vi "STC_main_raw_dev_MQTTT_RT_raw.vi"() -> ()   [LabVIEW 2017]
uses:
  controls/FPGA State.ctl
  mqtt Folder/src/class/mqtt/mqttTypedef/mqttConnectionStatus.ctl
  mqtt Folder/src/class/mqtt/mqttTypedef/mqttConnectionMeta.ctl
  mqtt Folder/src/class/mqtt/mqttTypedef/mqttQOSlevel.ctl
  controls/UI Data2.ctl
  mqtt Folder/src/class/mqtt/mqttTXqueue/mqttTXdataQueueFunction.ctl
  mqtt Folder/src/class/mqtt/mqttConfigFunction.ctl
  mqtt Folder/src/class/mqtt/mqttTypedef/mqttConnectionFlags.ctl
  mqtt Folder/src/class/mqtt/mqttTypedef/mqttWillInformation.ctl
  mqtt Folder/src/class/mqtt/mqttTypedef/mqttBroker.ctl
  controls/Chatter data.ctl
  Globals/Global - All UI Loop Stop.vi
  Globals/Global - UI Stream and Variable Connections.vi
  Globals/Global - Configuration Options.vi
  UI Error Handlers/support/User Event - Stop/User Event - Stop.lvlib
  UI Error Handlers/support/Message Queue/Message Queue.lvlib
  mqtt Folder/src/class/mqtt/mqtt.lvclass
panel:
  out "publishSuccess":bool=TRUE
  out "publishMessageID":u16 format="%02x"
  in  "connMeta":T1
  in  "topic":string="a/b"
  out "connStatus 2":T3
  out "success":bool
  out "sessionPresent 2":bool
  in  "error in (no error)":errorcluster
  out "tag acc":string
  out "tag spike":string
  out "string":string
  out "x .or. y?":bool
  out "resulting string":string
  out "Raw Waveform":waveform(dbl)[](graph)
  in  "Settings Tab":T4(tab)=enum."Data Monitoring"
  in  "Database_machine":string="Raw.Starrag_STC_1250_V1"
  in  "OK Button":bool
  in  "Tool Data File":path=path "K:/Core Research/Project Folders/AI Projects/AI3190 Digital Shop Floor Rollout/5 Software Files/Catapult/tool_path.txt"
  in  "Run Control":bool
  in  "Stop Control":bool
  in  "Max Acceleration Threshold (g)":sgl=0.03
  in  "In-cut Power Threshold":dbl=1.0
  in  "Controller Address":string="143.167.158.195"
  in  "Connect to Controller":bool
  out "Connected?":bool
  out "System Status":string
  in  "Save?":bool
  in  "Switch to Safe State":bool
  out "Current FPGA State":T5
  out "Tool Data":string="\n"
  in  "ODBC data source name":string="amrc_monitoring"
  in  "MT Connect Agent":string="http://amrcmtconnect.shef.ac.uk:5000/"
  in  "milliseconds to wait":u32=100
  in  "Machine":string="STC1250"
  out "Loop execution":u32
  out "output cluster":cluster{"G1 ":bool}
  out "Chatter?":bool
  out "Feed":dbl
  out "ACC  (grms)":T6(graph)
  out "Block of code being executed":string
  out "Program Name":string
  out "RPM":dbl
  out "STC Starrag":bool
  out "Force (grms)":T7(graph)
  out "Tool id":string
  out "Spindle Load":dbl[](graph)
  out "CPU Usage (%)":dbl[][](graph)
  out "Free Physical Memory or Largest Contiguous Memory (bytes)":dbl(graph)
  out "DMA FIFO Overflow?":bool
  in  "Exit":bool
  # "Acceleration Waveform for 0.5s"
  # "Connection Settings"
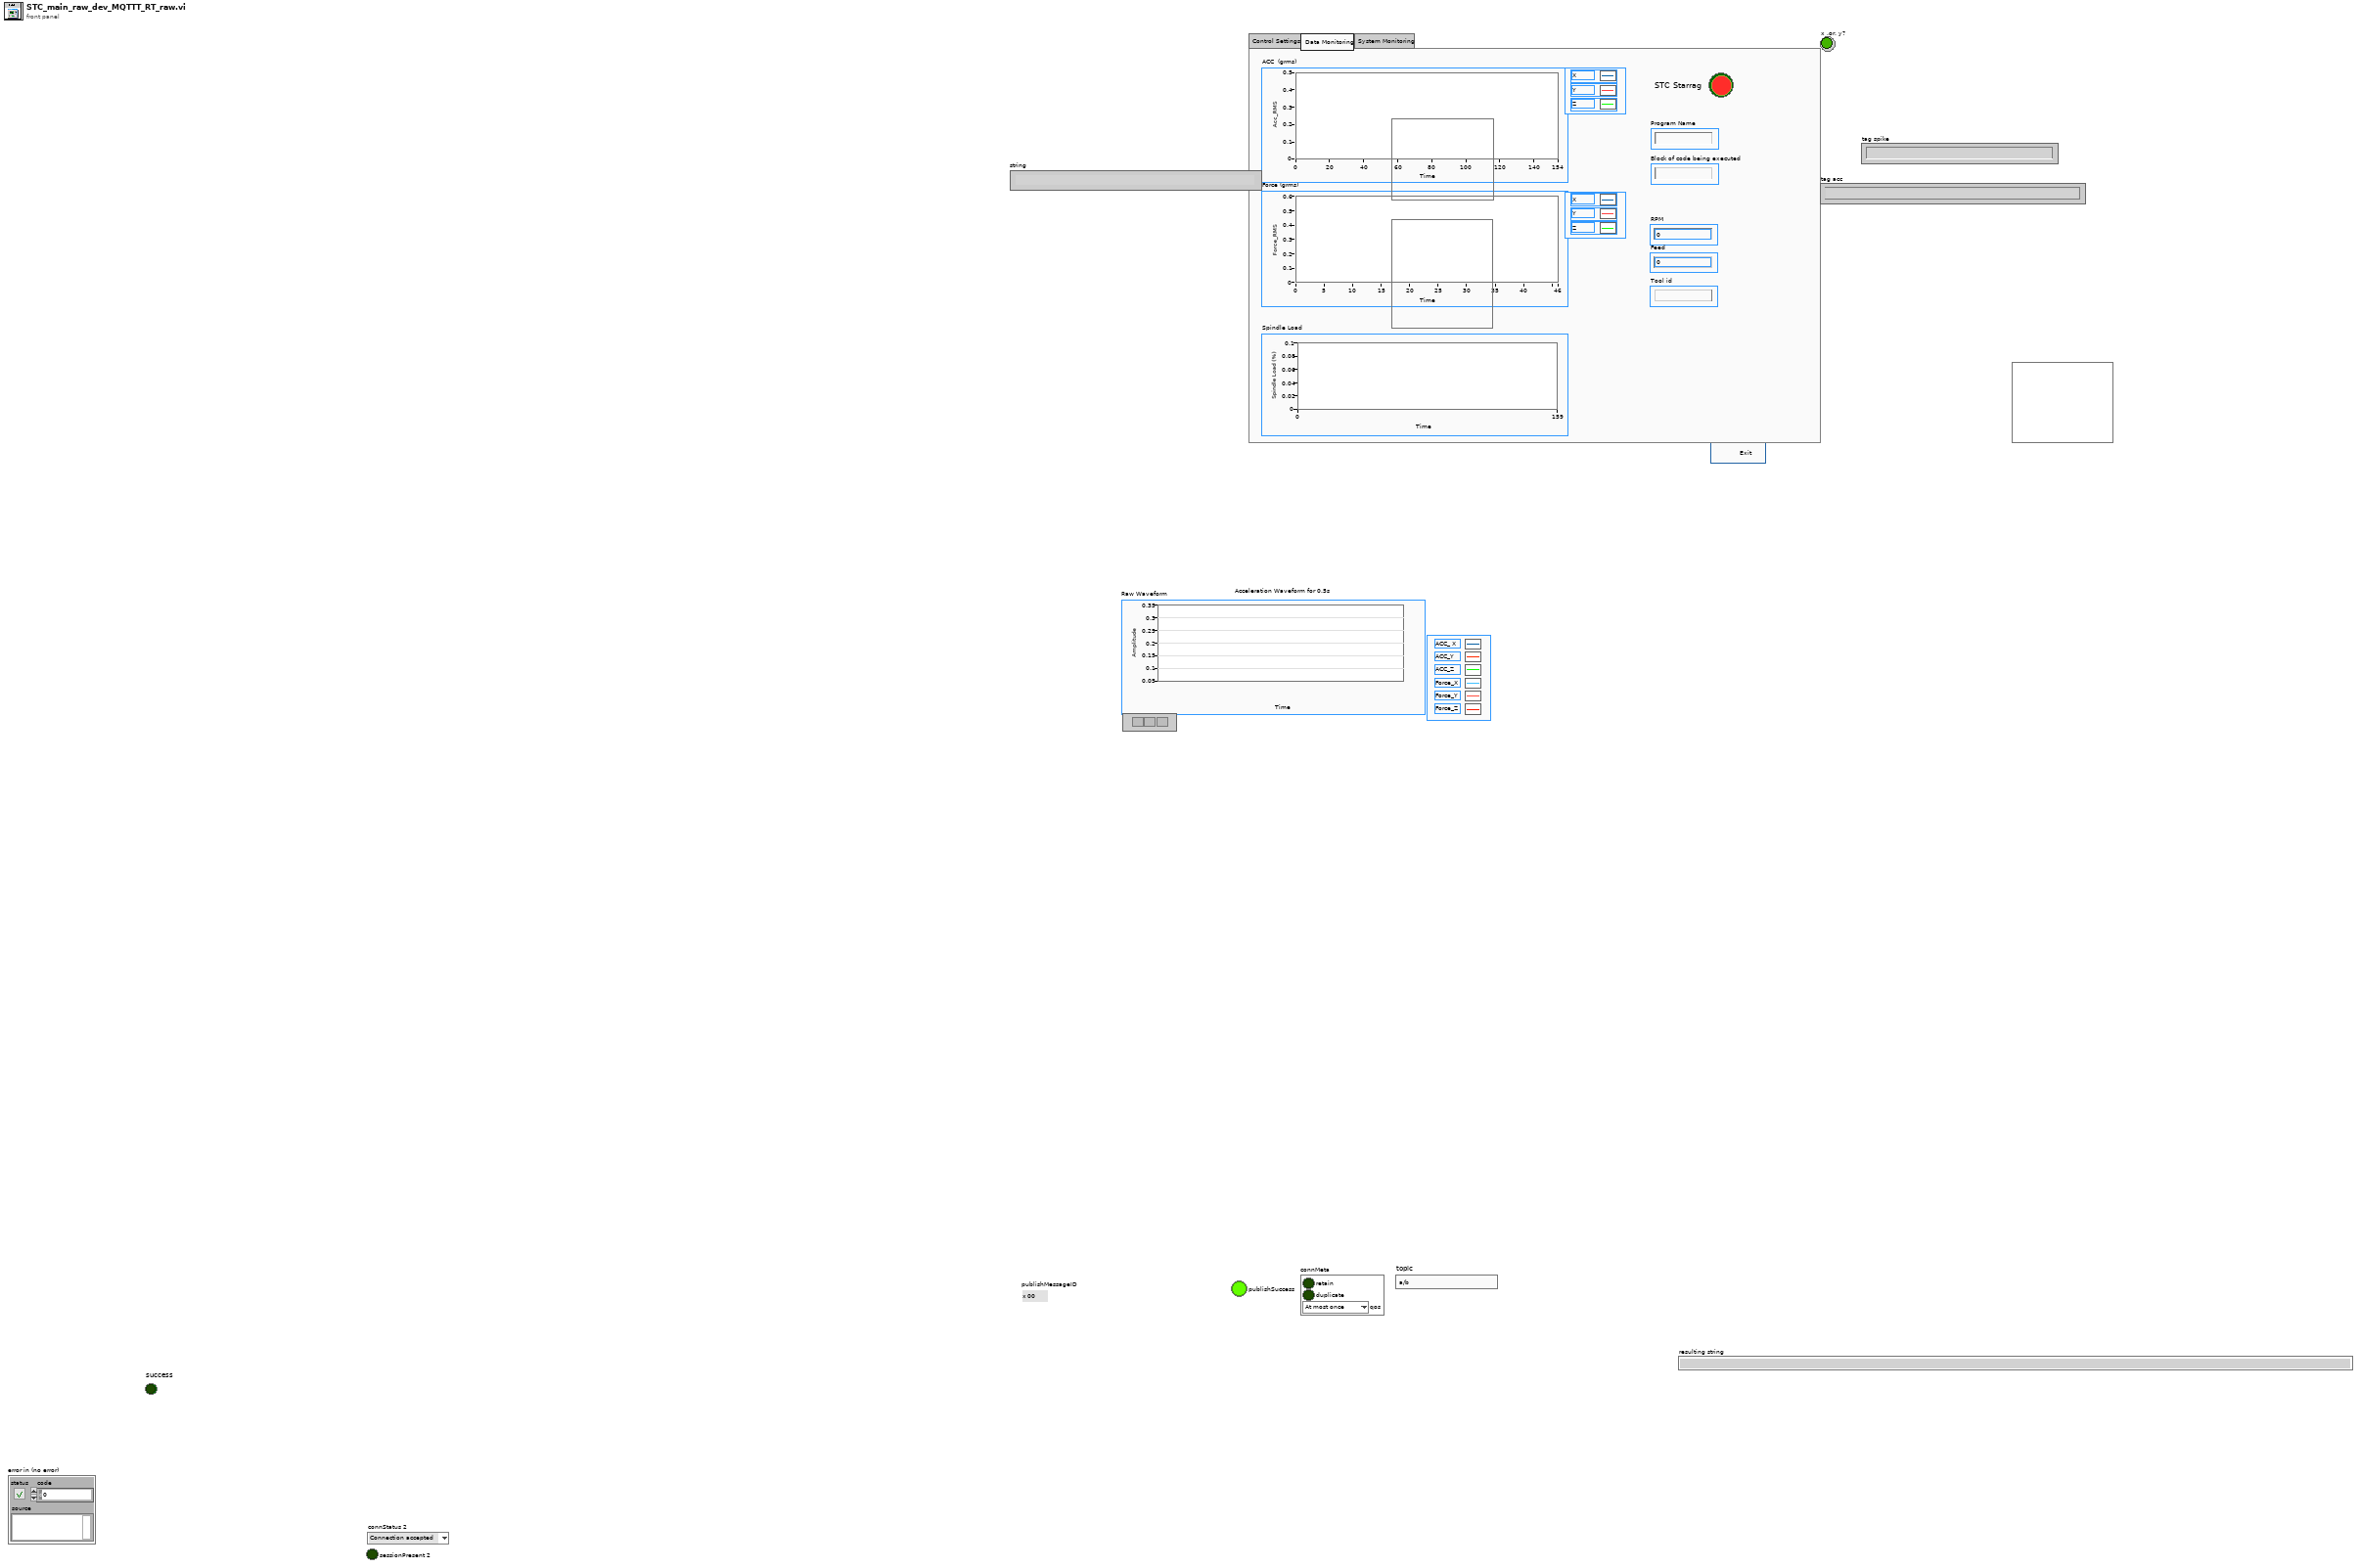
[diagram p1: front panel]
types:
  T1 = typedef "mqttConnectionMeta.ctl" = cluster{"retain":bool, "duplicate":bool, "qos":T2}
  T2 = typedef "mqttQOSlevel.ctl" = enum8{"At most once", "At least once", "Exactly once", "Reserved"}
  T3 = typedef "mqttConnectionStatus.ctl" = enum16{"Connection accepted", "Connection refused: unacceptable protocol version", "Connection refused: identifier rejected", "Connection refused: Server unavailable", "Connection refused: bad user name or password", "Connection refused: not authorized"}
  T4 = enum32{"Control Settings", "Data Monitoring", "System Monitoring"}
  T5 = typedef "FPGA State.ctl" = enum16{"Safe State", "Control (PID)"}
  T6 = cluster{"Array of Double[0]":dbl, "Array of Double[1]":dbl, "Array of Double[2]":dbl}
  T7 = cluster{"[0]":dbl, "[1]":dbl, "[2]":dbl, "[3]":dbl, "[4]":dbl, "[5]":dbl, "[6]":dbl, "[7]":dbl}
  T8 = typedef "mqttBroker.ctl" = cluster{"address":string, "port":u16, "connTimeout":i32, "writeTimeout":i32, "readTimeout":i32, "subTimeout":i32}
  T9 = typedef "mqttWillInformation.ctl" = cluster{"User Name":string, "Password":string}
  T10 = typedef "mqttConnectionFlags.ctl" = cluster{"reserved":bool, "clean session":bool, "will flag":bool, "willQOS":enum8{"At most once", "At least once", "Exactly once", "Reserved"}, "will retain":bool, "password":bool, "user name":bool}
  T11 = typedef "mqtt.lvclass/mqttConfigFunction.ctl" = enum16{"init", "deinit", "set", "get"}
  T12 = enum8{"Enabled", "Disabled", "Disabled and Grayed Out"}
  T13 = typedef "mqttTXdataQueueFunction.ctl" = enum16{"init", "deinit", "getQueue", "enqueue"}
  T14 = typedef "UI Data2.ctl" = cluster{"Switch to Safe State Ref":refnum<vi>, "Run Control Ref":refnum<vi>, "Stop Control Ref":refnum<vi>, "Update Control Configurations Ref":refnum<vi>, "Chatter Data Ref":refnum<vi>, "Max Acceleration Threshold Ref":refnum<vi>}
  T15 = typedef "Message Queue.lvlib/All Message Queues.ctl" = cluster{"UI":refnum<queue>}
  T16 = cluster{"Message":string, "Message Data":variant}
  T17 = typedef "Chatter data.ctl" = cluster{"Tool data":cluster{"Number of teeth":sgl}, "Cutting data":cluster{"rpm":sgl}, "Limits":cluster{"Magnitude threshold":sgl, "Tolerance":sgl}, "G1 status":cluster{"G1 ":bool}}
  T18 = cluster{"FPGA State":T5, "Max Acceleration Threshold":sgl, "Chatter Data":T17}
  T19 = cluster{"seconds since 1Jan1904":timestamp, "number":dbl[][], "Machine Data":cluster{"Zload":string, "Yload":string, "Xload":string, "path_position":string, "Fovr":string, "SspeedOvr":string, "Program Name":string, "Program status":string, "Block of code being executed":string, "Line of code":string, "Machine availability":string, "Emergency status":string, "Controller mode":string, "Tool_id":string}}
  T20 = cluster{"seconds since 1Jan1904":timestamp, "number":dbl[][], "Machine Data":cluster{"Zload":string, "Yload":string, "Xload":string, "path_position":string, "Fovr":string, "SspeedOvr":string, "Program Name":string, "Program status":string, "Block of code being executed":string, "Line of code":string, "Machine availability":string, "Emergency status":string, "Controller mode":string, "Tool id":string}}
  T21 = cluster{"Actual PID Loop Period":refnum<k21>, "DMA FIFO Overflow?":refnum<k21>, "CPU Usage":refnum<k21>, "Free or Contiguous Memory":refnum<k21>, "Current FPGA State":refnum<k21>, "Acceleration (grms)":refnum<k21>, "Acceleration Waveform":refnum<k21>, "Chatter":refnum<k21>, "tag acc":refnum<k21>, "tag video":refnum<k21>, "Image Waveform":refnum<k21>}
  T22 = cluster{"Zload":string, "Yload":string, "Xload":string, "path_position":string, "Fovr":string, "SspeedOvr":string, "Program Name":string, "Program status":string, "Block of code being executed":string, "Line of code":string, "Machine availability":string, "Emergency status":string, "Controller mode":string, "Tool_id":string}
  T23 = cluster{"Zload":string, "Yload":string, "Xload":string, "path_position":string, "Fovr":string, "SspeedOvr":string, "Program Name":string, "Program status":string, "Block of code being executed":string, "Line of code":string, "Machine availability":string, "Emergency status":string, "Controller mode":string, "Tool id":string}
  T24 = cluster{"Magnitude threshold":sgl, "Tolerance":sgl}
  T25 = typedef "FPGA state.ctl" = enum16{"Safe State", "Control (PID)"}
  T26 = typedef "IMAQ Image.ctl" = refnum<image>
  T27 = typedef "CPU Loads.ctl" = cluster{"Total (%)":dbl, "Time Critical (%)":dbl, "Timed Structures (%)":dbl, "High (%)":dbl, "Above Normal (%)":dbl, "Normal (%)":dbl, "Background (%)":dbl, "Idle (%)":dbl, "ISR (%)":dbl}[]
  T28 = cluster{"seconds since 1Jan1904":timestamp, "appended array":dbl[][], "Machine Data":cluster{"Zload":string, "Yload":string, "Xload":string, "path_position":string, "Fovr":string, "SspeedOvr":string, "Program Name":string, "Program status":string, "Block of code being executed":string, "Line of code":string, "Machine availability":string, "Emergency status":string, "Controller mode":string, "Tool_id":string}}
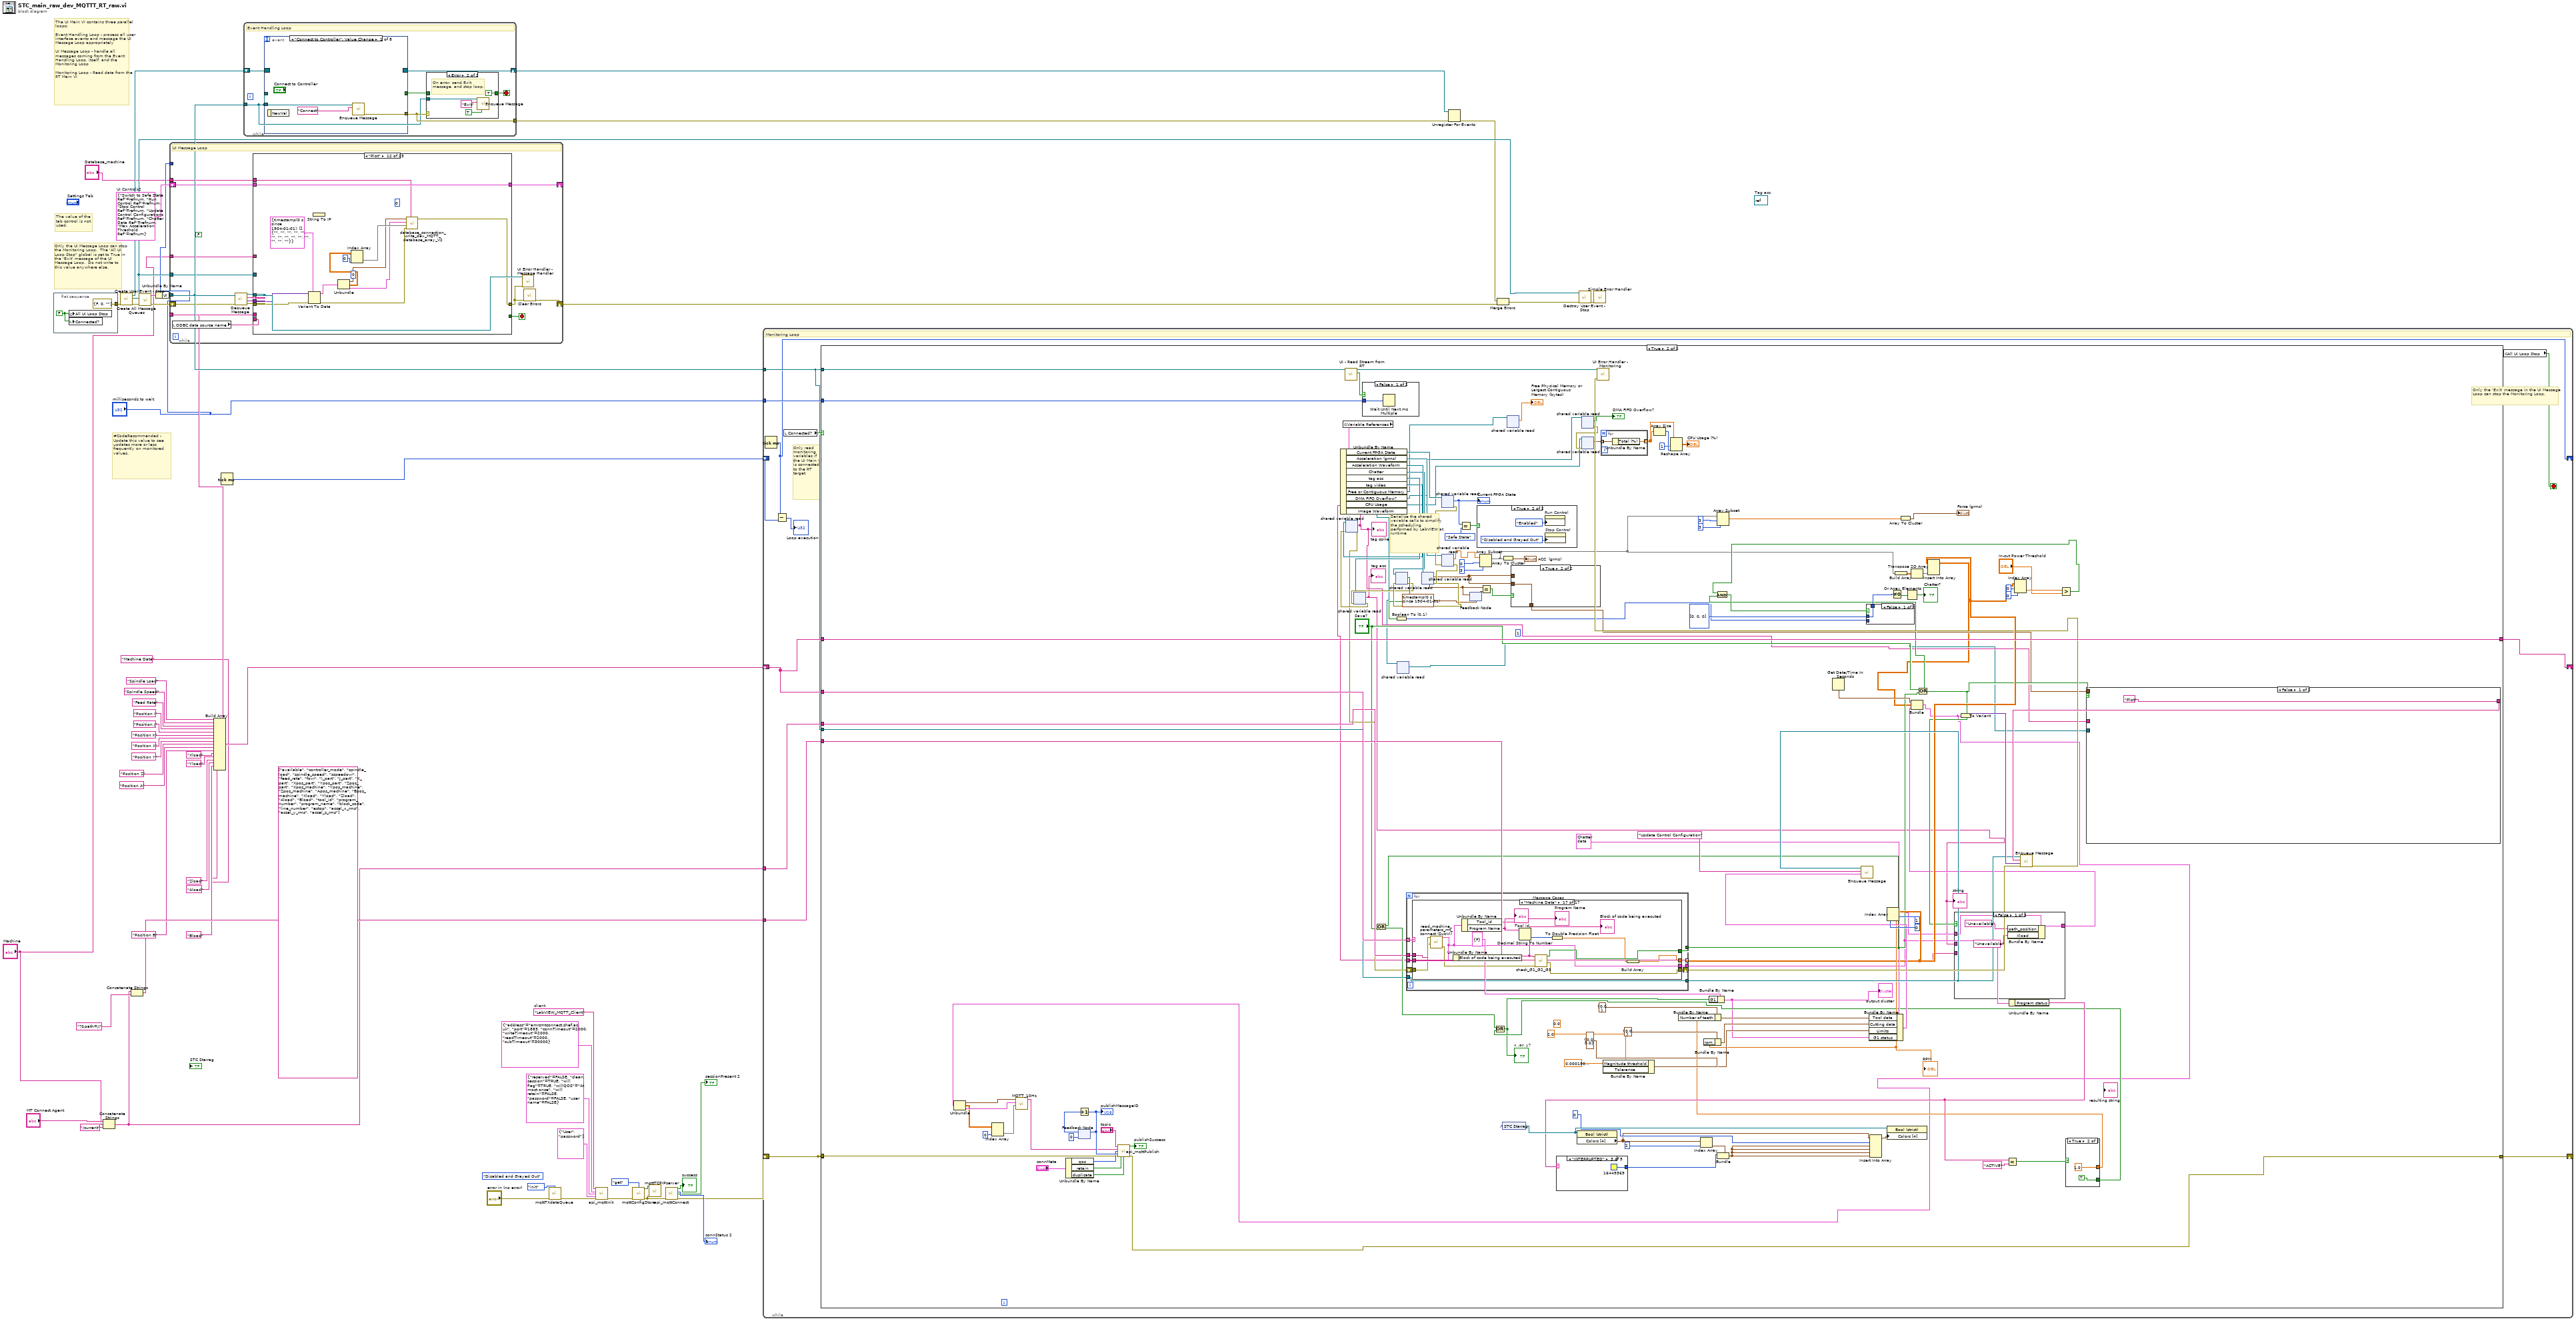
[diagram p0: block diagram]
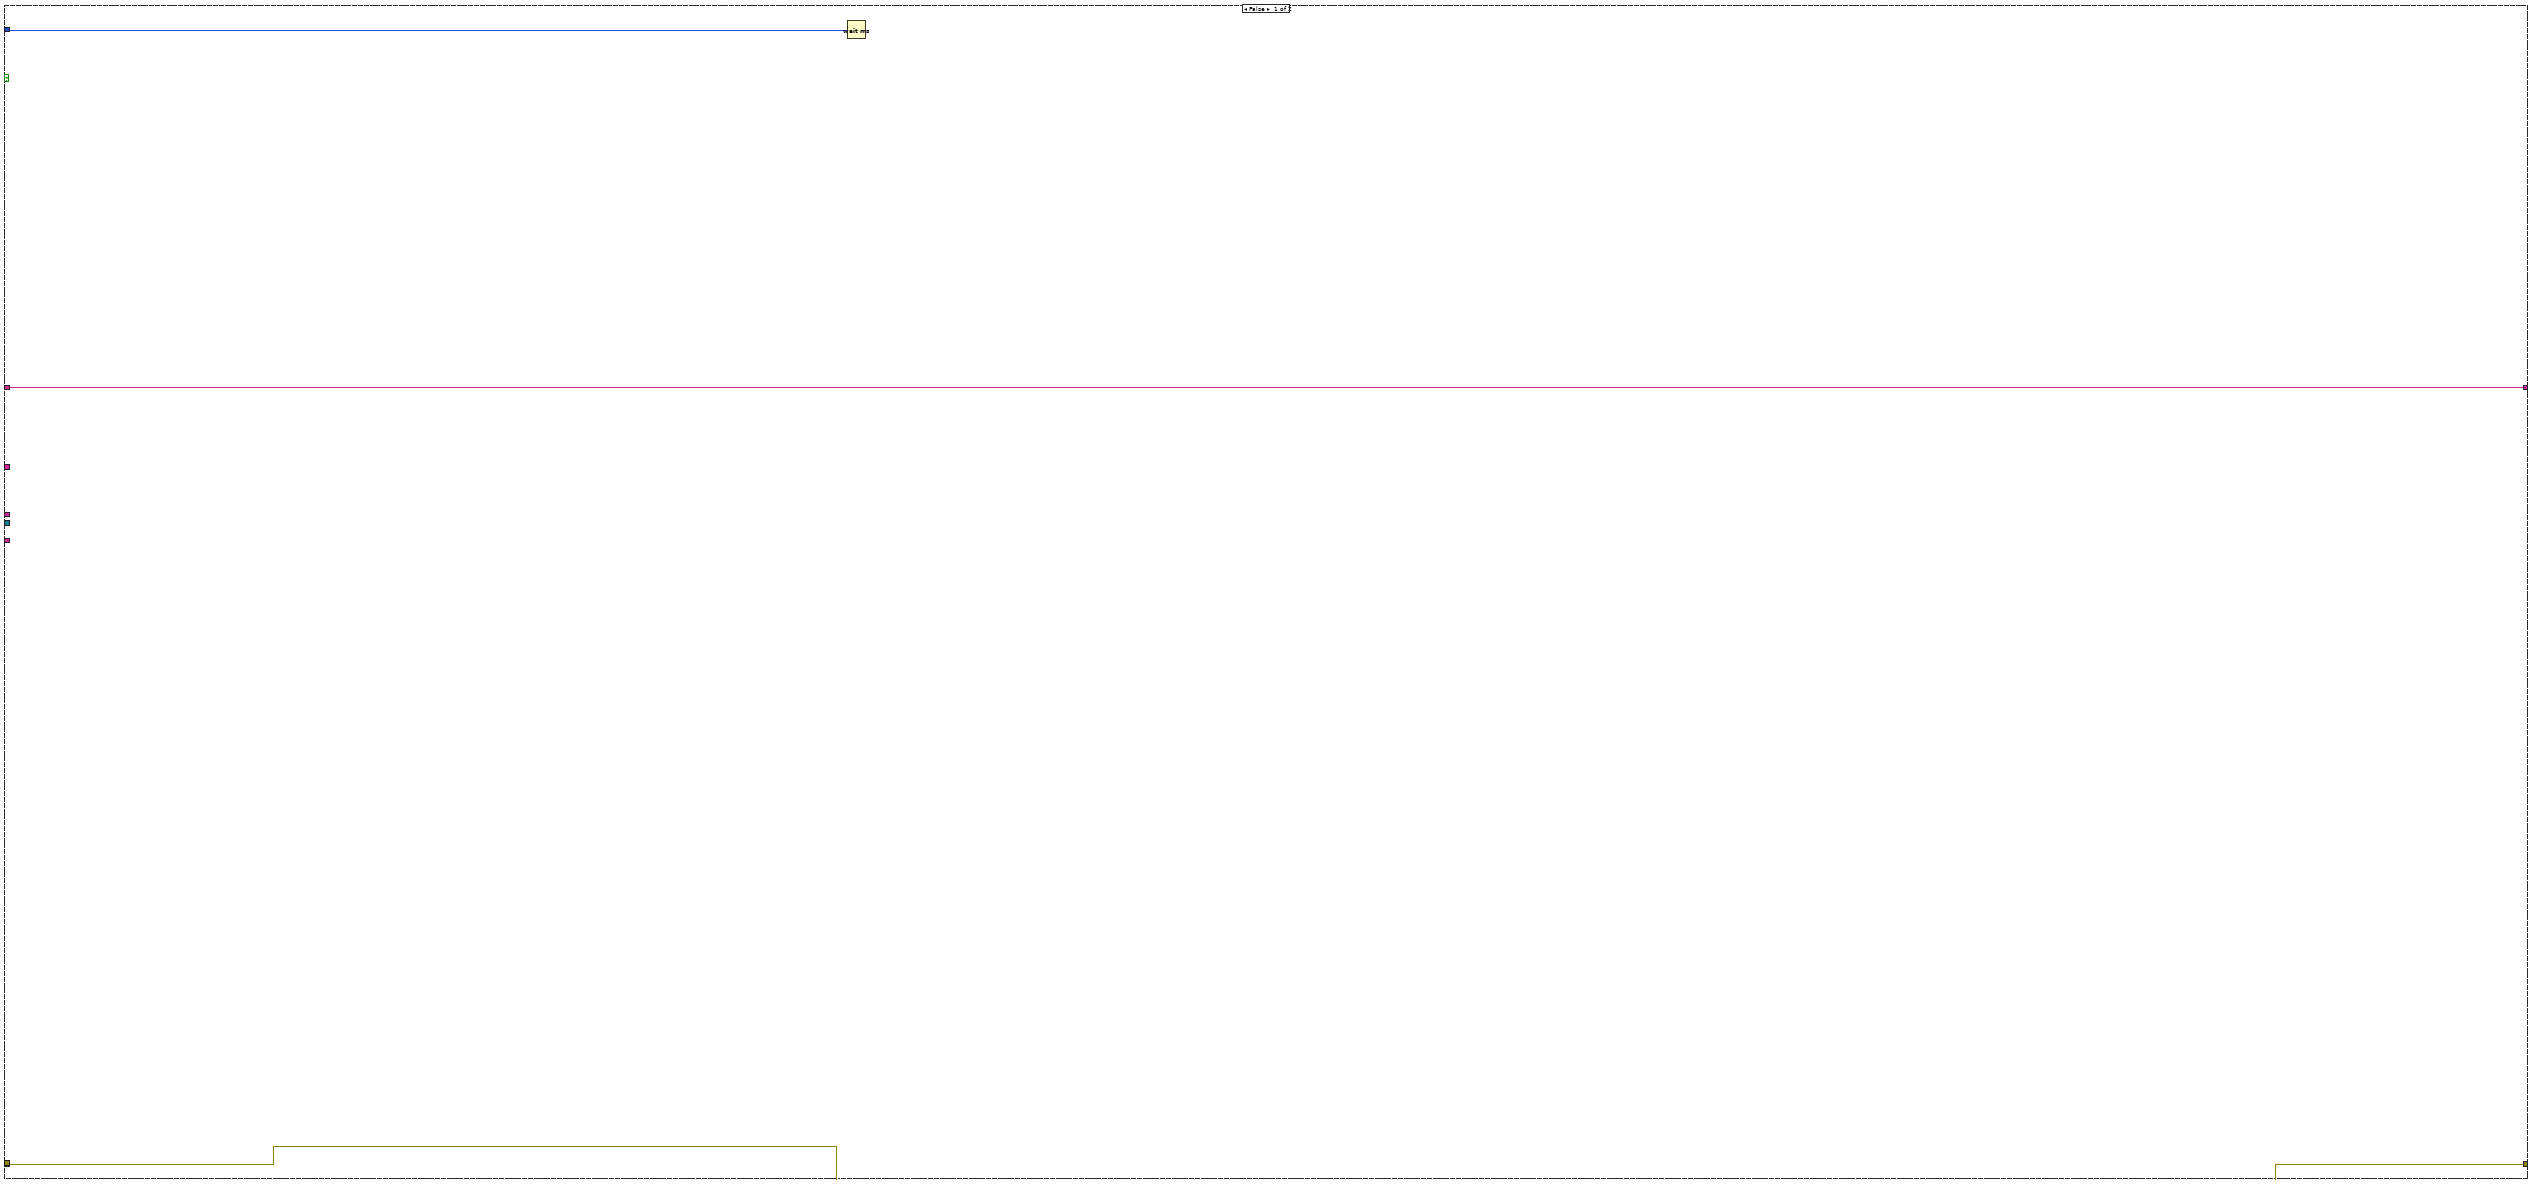
[diagram p2: hidden frame]
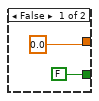
[diagram p3: hidden frame]
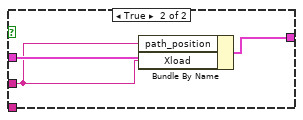
[diagram p4: hidden frame]
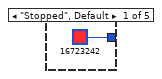
[diagram p5: hidden frame]
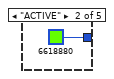
[diagram p6: hidden frame]
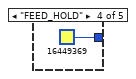
[diagram p7: hidden frame]
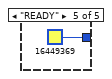
[diagram p8: hidden frame]
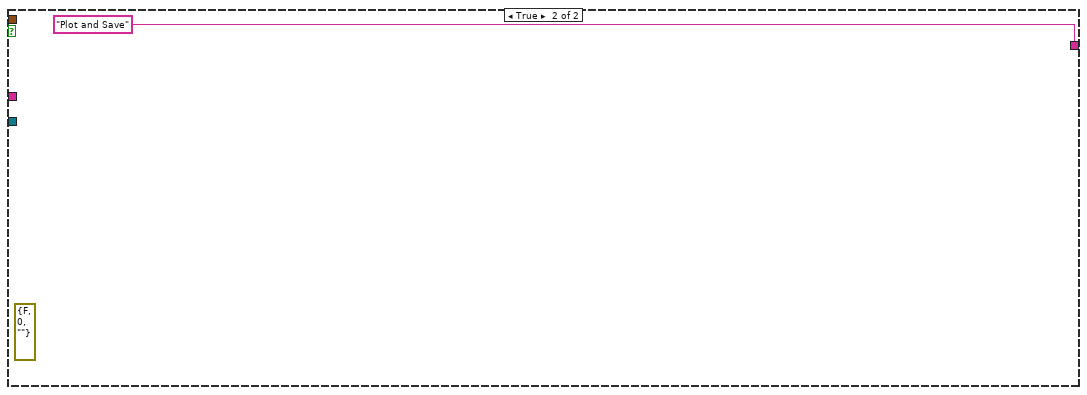
[diagram p10: hidden frame]
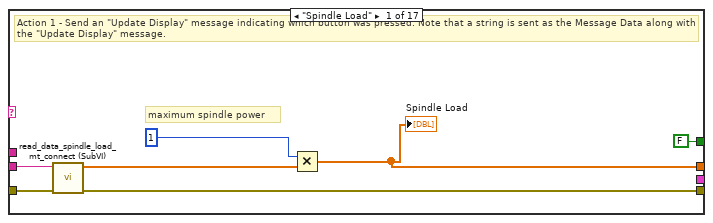
[diagram p11: hidden frame]
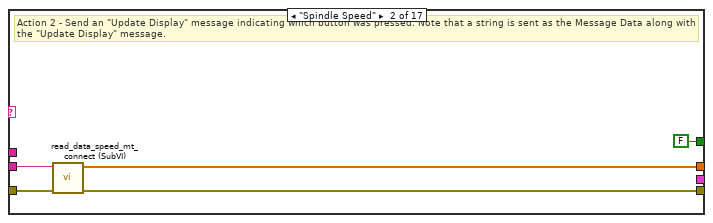
[diagram p12: hidden frame]
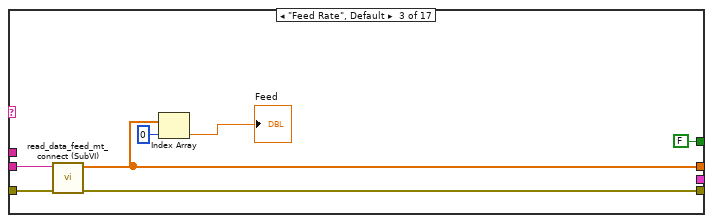
[diagram p13: hidden frame]
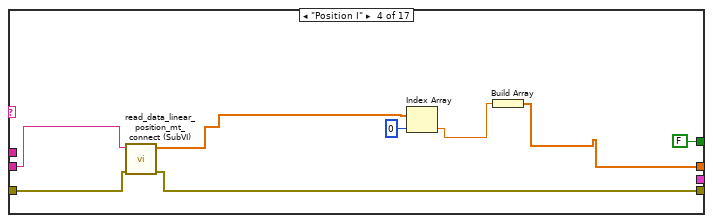
[diagram p14: hidden frame]
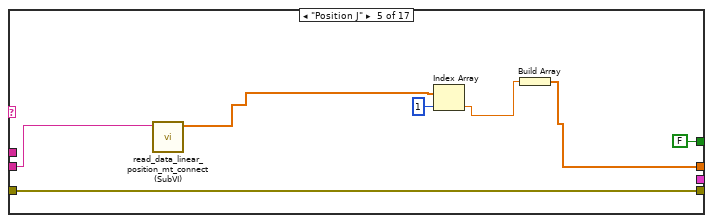
[diagram p15: hidden frame]
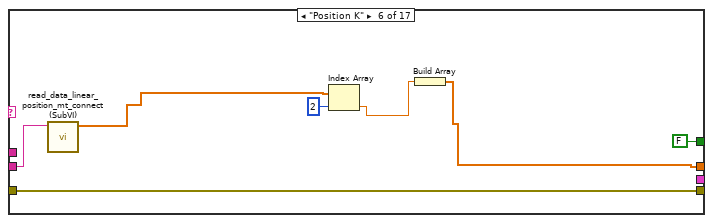
[diagram p16: hidden frame]
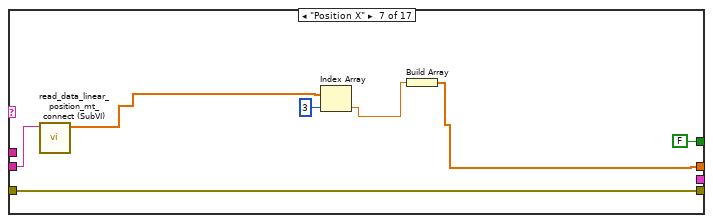
[diagram p17: hidden frame]
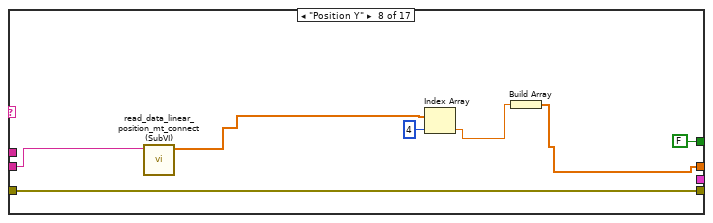
[diagram p18: hidden frame]
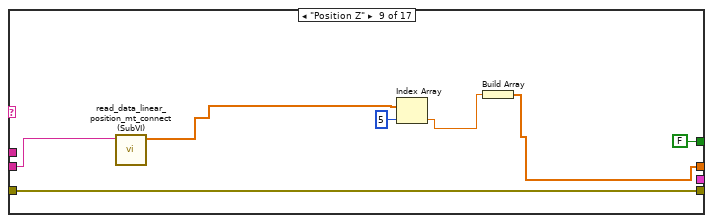
[diagram p19: hidden frame]
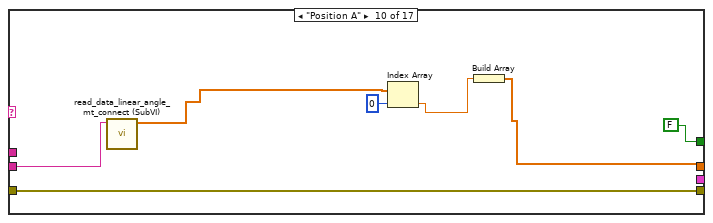
[diagram p20: hidden frame]
diagram:
  w6 = "LabVIEW_MQTT_Client"  # client
  (unwired) T12."Disabled and Grayed Out" ("Disabled")
  (unwired) string[] ["available", "controller_mode", "spindle_load", "spindle_speed", "sspeedovr", "feed_rate", "fovr", "I_part", "J_part", "K_part", "Xpos_part", "Ypos_part", "Zpos_part", "Xpos_machine", "Ypos_machine", "Zpos_machine", "Apos_machine", "Bpos_machine", "Xload", "Yload", "Zload", "Aload", "Bload", "tool_id", "program_number", "program_name", "block_code", "line_number", "estop", "accel_x_rms", "accel_y_rms", "accel_z_rms"]
  (unwired) refnum<k21> refnum  # Tag acc
  (unwired) FALSE ("Record  SS 661")
  w43 = T14 {"Switch to Safe State Ref"=refnum, "Run Control Ref"=refnum, "Stop Control Ref"=refnum, "Update Control Configurations Ref"=refnum, "Chatter Data Ref"=refnum, "Max Acceleration Threshold Ref"=refnum}  # UI Controls2
  # "#CodeRecommended - Update this value to see updates more or less frequently on monitored values."
  # "The UI Main VI contains three parallel loops:\n\nEvent Handling Loop - process all user interface events and message the UI Message Loop appropriately\n\nUI Message Loop - handle all messages coming from the Event Handling Loop, itself, and the Monitoring Loop\n\nMonitoring Loop - Read data from the RT Main VI"
  # "The value of the tab control is not used."
  # "Only the UI Message Loop can stop the Monitoring Loop.  The 'All UI Loop Stop\" global is set to True in the 'Exit' message of the UI Message Loop.  Do not write to this value anywhere else."
  n1 = flat-sequence {
    tunnel: [errorcluster {"status"=FALSE, "code"=0, "source"=""} ("error in (no error)")] -> w44
    frame #0 {
      w57 = FALSE
      n2 = global write "Global - All UI Loop Stop.vi" "All UI Loop Stop"(w57) -> ()
      n3 = local write "Connected?"(w57) -> ()
    }
  }
  n4 = Concatenate Strings("MT Connect Agent", "Machine", "/current" ("string")) -> (w34:string)
  n5 = call "Create User Event - Stop.vi"("error in (no error)"=w44) -> ("error out"=w51:errorcluster, "User Event - Stop"=w52:refnum<user-event>, "Stop Event Registration Refnum"=w53:refnum<event-registration>)  [unwired: 8 in]
  n6 = Concatenate Strings(w34, "?&path=//" ("string")) -> (w38:string)
  n7 = call "Create All Message Queues.vi"("error in (no error)"=w51) -> ("error out"=w49:errorcluster, "Message Queues out"=w50:T15)  [unwired: 9 in]
  n8 = Unbundle By Name(w50) -> ("UI"=w45:refnum<queue>)
  n9 = Build Array("Spindle Load" ("Message"), "Spindle Speed" ("Message"), "Feed Rate" ("element"), "Position I" ("element"), "Position J" ("element"), "Position K" ("element"), "Position X" ("element"), "Position Y" ("element"), "Position Z" ("element"), "Position A" ("element"), "Position B" ("element"), "Xload" ("element"), "Yload" ("element"), "Zload" ("element"), "Aload" ("element"), "Bload" ("element"), "Machine Data" ("element")) -> (w37:string[])
  n10 = while {
    tunnel: w45 -> [w68]
    tunnel: w52 -> [w73]
    shift-right: [w63] -> w56
    shift-left: w49 -> [w72]
    shift-right: [w66] -> _
    shift-left: w43 -> [w67]
    tunnel: w37 -> [w62]
    tunnel: "Machine" -> [w61]
    tunnel: "milliseconds to wait" -> [_]
    tunnel: "Database_machine" -> [w59]
    stop <- w74 stop-if-true
    # "UI Message Loop"
    n11 = local read "ODBC data source name"() -> (w60:string)
    n12 = call "Dequeue Message.vi"("error in (no error)"=w72, "Message Queue"=w68) -> ("error out"=w71:errorcluster, "Message Data"=w69:variant, "Message"=w70:string, "dup Message Queue"=w65:refnum<queue>)  [unwired: 6 in]
    n13 = case "Message Cases" shown="\"Plot\"" w70 {
      selector: w70 -> [_ _ _ _ _ _ _ _ _ _ _ _ w205 _ w239 _ w274 _ _ _ _ _ w373]
      tunnel: w65 -> [w76 w82 _ _ w115 _ w133 w141 _ w166 _ _ w206 _ _ _ w278 _ w321 _ _ w347 _]
      tunnel: w71 -> [w78 w89 w102 w108 w120 w131 w135 w139 w155 w175 w189 w202 w208 w226 w240 w258 w288 w309 w326 w331 w343 w348 _]
      tunnel: [w77 w83 w102 w108 w114 w131 w134 w144 w154 w168 w182 w194 w207 w228 w241 w257 w289 w307 w327 w330 w342 w351 w371] -> w64
      tunnel: [_ _ _ _ _ _ _ _ _ _ _ _ _ _ _ _ _ _ TRUE _ _ _ _] -> w74
      tunnel: w69 -> [_ _ _ _ _ _ _ _ _ w173 w188 w201 _ w225 w238 w256 w286 w306 _ _ w340 _ _]
      tunnel: w73 -> [_ _ _ _ _ _ _ _ _ _ _ _ _ _ _ _ _ _ w325 _ _ _ _]
      tunnel: w67 -> [w79 w88 w101 w110 w119 w130 w137 w145 w156 w171 w190 w203 w209 w229 w242 w255 w290 w308 w323 w329 w341 w350 w369]
      tunnel: [w79 w87 w101 w110 w119 w130 w137 w145 w156 w171 w190 w203 w209 w229 w242 w255 w290 w308 w323 w329 w341 w350 w369] -> w66
      tunnel: w62 -> [_ _ _ _ _ _ _ _ _ _ _ _ _ _ _ _ _ _ _ _ _ _ _]
      tunnel: w60 -> [_ _ _ _ _ _ _ _ _ _ _ _ _ _ _ _ _ _ _ _ _ _ _]
      tunnel: w61 -> [_ _ _ _ _ _ _ _ _ _ _ _ _ _ _ _ _ _ _ _ _ _ _]
      tunnel: w59 -> [_ _ _ _ _ _ _ _ _ _ w178 w191 _ _ _ _ _ _ _ _ _ _ _]
      frame "Initialize" {
        # "Initialize - Send 'Initialize UI Refs' message to get the UI references bundled and initialized appropriately."
        n14 = call "Enqueue Message.vi"("error in (no error)"=w78, "Message"="Initialize UI Refs", "Message Queue"=w76) -> ("error out"=w77:errorcluster)  [unwired: 7 in, 1 out]
      }
      frame "Initialize UI Refs" {
        # "Send a message to disable them all, since there is no connection at the start."
        # "Initialize UI Refs - Bundle up a cluster of references of all UI elements that are programmatically manipulated."
        n15 = control-ref of="Max Acceleration Threshold (g)"() -> (w80:refnum<vi>)
        n16 = control-ref of="Switch to Safe State"() -> (w86:refnum<vi>)
        n17 = control-ref of="Run Control"() -> (w85:refnum<vi>)
        n18 = control-ref of="Stop Control"() -> (w84:refnum<vi>)
        n19 = call "Enqueue Message.vi"("error in (no error)"=w89, "Message"="Disable Controls", "Message Queue"=w82) -> ("error out"=w83:errorcluster)  [unwired: 7 in, 1 out]
        n20 = Bundle By Name(cluster=w88, "Switch to Safe State Ref"=w86, "Run Control Ref"=w85, "Stop Control Ref"=w84, "Max Acceleration Threshold Ref"=w80) -> (w87:T14)
      }
      frame "Disable Controls" {
        w92 = 0
        # "With the control options disabled, the only thing the user can do is Connect. Make sure the IP address string and connect button are enabled."
        # "Disable All Controls - Set all controls in the UI Refs cluster to \"Disabled and Grayed Out\"."
        n21 = Unbundle(w101) -> ("Switch to Safe State Ref"=w100:refnum<vi>, "Run Control Ref"=w99:refnum<vi>, "Stop Control Ref"=w98:refnum<vi>, "Update Control Configurations Ref"=w97:refnum<vi>, "Chatter Data Ref"=w96:refnum<vi>, "Max Acceleration Threshold Ref"=w95:refnum<vi>)
        n22 = Build Array(w100, w99, w98, w97, w96, w95) -> (w94:refnum<vi>[])
        n23 = property on="ODBC data source name" class="Str"("DisabledEnum"=T12."Enabled" ("Disabled")) -> ()  [unwired: 2 in, 2 out]
        n24 = property on="In-cut Power Threshold" class="DigNum (strict)"("DisabledEnum"=T12."Disabled and Grayed Out" ("Disabled")) -> ()  [unwired: 2 in, 2 out]
        n25 = call "Set Enable State on Multiple Controls.vi"("Enable?"=FALSE, "Controls"=w94) -> ()  [unwired: 10 in]
        n26 = property on="Controller Address" class="Str"("DisabledEnum"=w92) -> ()  [unwired: 2 in, 2 out]
        n27 = property on="Connect to Controller" class="Bool"("DisabledEnum"=w92) -> ()  [unwired: 2 in, 2 out]
      }
      frame "Enable Configuration Controls" {
        w111 = 2
        # "Once connected, the user shouldn't be able to change the connection settings unless he gets disconnected."
        # "Enable Configuration Controls - After successful connection, ensure appropriate controls are enabled."
        n28 = Unbundle By Name(w110) -> ("Update Control Configurations Ref"=w109:refnum<vi>, "Max Acceleration Threshold Ref"=w107:refnum<vi>, "Chatter Data Ref"=w106:refnum<vi>, "Switch to Safe State Ref"=w105:refnum<vi>)
        n29 = property on="In-cut Power Threshold" class="DigNum (strict)"("DisabledEnum"=T12."Enabled" ("Disabled")) -> ()  [unwired: 2 in, 2 out]
        n30 = property on="ODBC data source name" class="Str"("DisabledEnum"=T12."Disabled and Grayed Out" ("Disabled")) -> ()  [unwired: 2 in, 2 out]
        n31 = Build Array(w109, w107, w106, w105) -> (w113:refnum<vi>[])
        n32 = call "Set Enable State on Multiple Controls.vi"("Enable?"=TRUE, "Controls"=w113) -> ()  [unwired: 10 in]
        n33 = property on="Controller Address" class="Str"("DisabledEnum"=w111) -> ()  [unwired: 2 in, 2 out]
        n34 = property on="Connect to Controller" class="Bool"("DisabledEnum"=w111) -> ()  [unwired: 2 in, 2 out]
      }
      frame "Connect" {
        # "Connect - Attempt to connect to both streams, and the variables, on the RT target."
        n35 = call "UI - Initiate Connection.vi"("error in (no error)"=w120, "Controller Address"="Controller Address", "Message Queue"=w115) -> ("error out"=w117:errorcluster, "Connected?"=w116:bool)  [unwired: 7 in]
        "Connected?" <- w116
        n36 = case shown="True" w116 {
          tunnel: w117 -> [w121 w125]
          tunnel: w115 -> [_ w124]
          tunnel: [w121 w123] -> w114
          frame False {
          }
          frame True {
            n37 = call "Enqueue Message.vi"("error in (no error)"=w125, "Message"="Enable Configuration Controls", "Message Queue"=w124) -> ("error out"=w123:errorcluster)  [unwired: 7 in, 1 out]
          }
        }
      }
      frame "Close Connections" {
        # "Close Connections - Close the connections shared with the Monitoring Loop."
        n38 = global read "Global - UI Stream and Variable Connections.vi" "UI Command Stream"() -> (w129:refnum<k21>)
        n39 = global read "Global - UI Stream and Variable Connections.vi" "RT Message Stream"() -> (w128:refnum<k21>)
        n40 = global read "Global - UI Stream and Variable Connections.vi" "Variable References"() -> (w126:T21)
        n41 = local write "Connected?"(FALSE ("Connected?")) -> ()
        n42 = Destroy Stream Endpoint(11:w129) -> ()  [unwired: 1 in, 1 out]
        n43 = Destroy Stream Endpoint(11:w128) -> ()  [unwired: 1 in, 1 out]
        n44 = call "Close Variable Connections.vi"("Variable References 2"=w126) -> ()  [unwired: 11 in]
      }
      frame "Disconnect UI" {
        # "Disable Controls"
        # "Disconnect UI - Something has gone wrong with the connection. Reinitialize the UI to its disconnected state."
        n45 = local write "Connected?"(FALSE ("Connected?")) -> ()
        n46 = call "Enqueue Message.vi"("error in (no error)"=w135, "Message"="Reconnect", "Message Queue"=w133) -> ("error out"=w134:errorcluster)  [unwired: 7 in, 1 out]
      }
      frame "Reconnect" {
        # "Disconnect UI - Something has gone wrong with the connection. Reinitialize the UI to its disconnected state."
        n47 = Flush Queue(queue=w141, error in (no error)=w139) -> (queue out=w140:refnum<queue>, error out=w138:errorcluster)  [unwired: 1 out]
        n48 = flat-sequence {
          tunnel: w140 -> [w147]
          tunnel: w138 -> [w148]
          tunnel: [w148] -> w143
          tunnel: [w147] -> w142
          tunnel: w143 -> [w151]
          tunnel: w142 -> [w149]
          tunnel: [w150] -> w144
          frame #0 {
            n49 = Wait Until Next ms Multiple(millisecond multiple=u32 10000) -> ()  [unwired: 1 out]
          }
          frame #1 {
            n50 = call "Enqueue Message.vi"("error in (no error)"=w151, "Message"="Connect", "Message Queue"=w149) -> ("error out"=w150:errorcluster)  [unwired: 7 in, 1 out]
          }
        }
      }
      frame "Get Settings from FPGA" {
        # "Get Settings from FPGA - Send a command to the RT to retrieve all current FPGA Main VI parameter values and send them back to the UI."
        n51 = local read "Connected?"() -> (w153:bool)
        n52 = case shown="True" w153 {
          tunnel: w155 -> [w157 w161]
          tunnel: [w157 w160] -> w154
          frame False {
            # "Don't bother trying to send a message to the RT system if UI Main VI isn't even connected"
          }
          frame True {
            n53 = global read "Global - UI Stream and Variable Connections.vi" "UI Command Stream"() -> (w158:refnum<k21>)
            n54 = shared-variable-write(w158, w161, T16 {"Message"="Send FPGA Configuration to UI", "Message Data"=variant} ("data in")) -> (w160:errorcluster)  [unwired: 1 in, 2 out]
          }
        }
      }
      frame "Initial UI Values" {
        # "Set values of all manual and setpoint controls via reference."
        # "Initial UI Values - These are the current values of the FPGA Main VI's R/W controls. They are used to initialize the panel of UI Main VI upon successful connection to the RT target."
        n55 = Variant To Data(error in=w175, type=T18 {"FPGA State"=enum."Safe State", "Max Acceleration Threshold"=0.0, "Chatter Data"={"Tool data"={"Number of teeth"=2.0}, "Cutting data"={"rpm"=9898.0}, "Limits"={"Magnitude threshold"=0.0, "Tolerance"=1.0}, "G1 status"={"G1 "=FALSE}}}, Variant=w173) -> (data=w172:T18, error out=w174:errorcluster)
        n56 = Unbundle By Name(w171) -> ("Max Acceleration Threshold Ref"=w163:refnum<vi>)
        n57 = Unbundle By Name(w172) -> ("Max Acceleration Threshold"=w165:sgl, "FPGA State"=w164:T5)  [unwired: 1 out]
        n58 = Build Array(w163, w163) -> (w170:refnum<vi>[])
        n59 = Build Array(w165) -> (w169:sgl[])
        n60 = for {
          tunnel: w170 -> [w177] mode=indexing
          tunnel: w169 -> [w176] mode=indexing
          n61 = property class="DigNum (strict)"(reference=w177, "Value"=w176) -> ()  [unwired: 1 in, 2 out]
        }
        n62 = local write "Current FPGA State"(w164) -> ()
        n63 = call "Enqueue Message.vi"("error in (no error)"=w174, "Message Data"=w164, "Message"="Update Display Mode", "Message Queue"=w166) -> ("error out"=w168:errorcluster)  [unwired: 6 in, 1 out]
      }
      frame "Plot and Save" {
        (unwired) u32 1 ("G1?")
        n64 = Variant To Data(error in=w189, type=T19 {"seconds since 1Jan1904"=timestamp(0 s since 1904-01-01), "number"=[], "Machine Data"={"Zload"="", "Yload"="", "Xload"="", "path_position"="", "Fovr"="", "SspeedOvr"="", "Program Name"="", "Program status"="", "Block of code being executed"="", "Line of code"="", "Machine availability"="", "Emergency status"="", "Controller mode"="", "Tool_id"=""}} ("output cluster"), Variant=w188) -> (data=w187:T19, error out=w179:errorcluster)
        n65 = Unbundle(w187) -> ("seconds since 1Jan1904"=w180:timestamp, "number"=w185:dbl[][], "Machine Data"=w183:T22)
        n66 = Index Array(array=w185, index (col)=0 ("disabled index (col)")) -> (element=w181:dbl[])  [unwired: 1 in]
        n67 = call "database_connection_write_dev_MQTT_database_array_V2.vi"("string"=w178, "error in (no error)"=w179, "data 2"=w181, "Machine Data"=w183, "current time 2"=w180) -> ("error out"=w182:errorcluster)  [unwired: 6 in]
      }
      frame "Plot" {
        (unwired) u32 0 ("G1?")
        (unwired) u32 0 ("G1?")
        n68 = Variant To Data(error in=w202, type=T20 {"seconds since 1Jan1904"=timestamp(0 s since 1904-01-01), "number"=[], "Machine Data"={"Zload"="", "Yload"="", "Xload"="", "path_position"="", "Fovr"="", "SspeedOvr"="", "Program Name"="", "Program status"="", "Block of code being executed"="", "Line of code"="", "Machine availability"="", "Emergency status"="", "Controller mode"="", "Tool id"=""}} ("output cluster"), Variant=w201) -> (data=w199:T20, error out=w192:errorcluster)
        n69 = String To IP() -> ()  [unwired: 1 in, 1 out]
        n70 = Unbundle(w199) -> ("seconds since 1Jan1904"=w193:timestamp, "number"=w197:dbl[][], "Machine Data"=w195:T23)
        n71 = Index Array(array=w197, index (col)=0 ("disabled index (col)")) -> (element=w196:dbl[])  [unwired: 1 in]
        n72 = call "database_connection_write_dev_MQTT_database_array_V2.vi"("string"=w191, "error in (no error)"=w192, "data 2"=w196, "Machine Data"=w195, "current time 2"=w193) -> ("error out"=w194:errorcluster)  [unwired: 6 in]
      }
      frame "Run Control", "Run Safe State", "Stop Control" {
        # "Run/Stop buttons - Send a command to switch the FPGA into the appropriate state. Send a message to update this UI to reflect the new state."
        n73 = local read "Connected?"() -> (w204:bool)
        n74 = case shown="False" w204 {
          tunnel: w208 -> [w210 w220]
          tunnel: [w210 w216] -> w207
          tunnel: w206 -> [_ w215]
          tunnel: w205 -> [_ w214]
          frame False {
            # "Don't bother trying to send a message to the RT system if UI Main VI isn't even connected"
          }
          frame True {
            # "Run Control switch into Run Control state. Anything else switches to Safe State."
            n75 = case shown="\"Run Control\"" w214 {
              tunnel: [FPGA_State."Safe State" ("FPGA State") FPGA_State."Control (PID)" ("FPGA State")] -> w211
              frame "Safe State", "Stop Control", Default {
              }
              frame "Run Control" {
              }
            }
            n76 = global read "Global - UI Stream and Variable Connections.vi" "UI Command Stream"() -> (w212:refnum<k21>)
            n77 = Bundle("Update FPGA State", "FPGA State"=w211) -> (w217:cluster{string, "FPGA State":T5})  [unwired: 1 in]
            n78 = shared-variable-write(w212, w220, w217) -> (w219:errorcluster)  [unwired: 1 in, 2 out]
            n79 = call "Enqueue Message.vi"("error in (no error)"=w219, "Message Data"=w211, "Message"="Update Display Mode", "Message Queue"=w215) -> ("error out"=w216:errorcluster)  [unwired: 6 in, 1 out]
          }
        }
      }
      frame "Update Control Configuration" {
        # "Update Control Configuration - Send all control configurations to RT to be sent down to the FPGA."
        n80 = Variant To Data(type=T17 {"Tool data"={"Number of teeth"=2.0}, "Cutting data"={"rpm"=9898.0}, "Limits"={"Magnitude threshold"=0.0, "Tolerance"=1.0}, "G1 status"={"G1 "=FALSE}} ("Chatter Data"), Variant=w225) -> (data=w224:T17)  [unwired: 1 in, 1 out]
        n81 = local read "Connected?"() -> (w227:bool)
        n82 = case shown="True" w227 {
          tunnel: w226 -> [w230 w236]
          tunnel: [w230 w235] -> w228
          tunnel: w224 -> [_ w231]
          frame False {
            # "Don't bother trying to send a message to the RT system if UI Main VI isn't even connected"
          }
          frame True {
            n83 = global read "Global - UI Stream and Variable Connections.vi" "UI Command Stream"() -> (w232:refnum<k21>)
            n84 = Bundle("Update Control Configurations", "Chatter Data"=w231) -> (w233:cluster{string, "Chatter Data":T17})  [unwired: 1 in]
            n85 = shared-variable-write(w232, w236, w233) -> (w235:errorcluster)  [unwired: 1 in, 2 out]
          }
        }
      }
      frame "Update Max Acceleration Threshold", "Update Max Fan Speed Threshold", "Update Setpoints" {
        # "Update Manual Values/Setpoints - Send all manual values/setpoints to RT to be sent down to the FPGA."
        n86 = local read "Connected?"() -> (w237:bool)
        n87 = case shown="True" w237 {
          tunnel: [w243 w249] -> w241
          tunnel: w240 -> [w243 w247]
          tunnel: w239 -> [_ w246]
          tunnel: w238 -> [_ w245]
          frame False {
            # "Don't bother trying to send a message to the RT system if UI Main VI isn't even connected"
          }
          frame True {
            n88 = global read "Global - UI Stream and Variable Connections.vi" "UI Command Stream"() -> (w244:refnum<k21>)
            n89 = Bundle(w246, "Message Data"=w245) -> (w248:cluster{string, "Message Data":variant})  [unwired: 1 in]
            n90 = shared-variable-write(w244, w247, w248) -> (w249:errorcluster)  [unwired: 1 in, 2 out]
          }
        }
      }
      frame "Update Display Mode" {
        # "Update Display Mode - Enable/Disable Controls appropriately for the new display mode."
        n91 = Variant To Data(error in=w258, type=FPGA_State."Safe State" ("FPGA State"), Variant=w256) -> (data=w254:T5, error out=w257:errorcluster)
        n92 = Unbundle By Name(w255) -> ("Switch to Safe State Ref"=w253:refnum<vi>, "Stop Control Ref"=w251:refnum<vi>, "Run Control Ref"=w250:refnum<vi>)
        n93 = case shown="\"Control (PID)\"" w254 {
          tunnel: w253 -> [w261 w267]
          tunnel: w250 -> [w259 w268]
          tunnel: w251 -> [w260 w266]
          frame "Control (PID)" {
            n94 = Build Array "Controls to Enable"(w261, w260) -> (w265:refnum<vi>[])
            n95 = Build Array "Controls to Disable"(w259) -> (w263:refnum<vi>[])
            n96 = call "Set Enable State on Multiple Controls.vi"("Enable?"=FALSE, "Controls"=w263) -> ()  [unwired: 10 in]
            n97 = call "Set Enable State on Multiple Controls.vi"("Enable?"=TRUE, "Controls"=w265) -> ()  [unwired: 10 in]
          }
          frame "Safe State", Default {
            # "This frame runs when FPGA is in Safe State. Only enable the run button."
            n98 = Build Array "Controls to Enable"(w268) -> (w272:refnum<vi>[])
            n99 = Build Array "Controls to Disable"(w267, w266) -> (w270:refnum<vi>[])
            n100 = call "Set Enable State on Multiple Controls.vi"("Enable?"=FALSE, "Controls"=w270) -> ()  [unwired: 10 in]
            n101 = call "Set Enable State on Multiple Controls.vi"("Enable?"=TRUE, "Controls"=w272) -> ()  [unwired: 10 in]
          }
        }
      }
      frame "Critical Error", "Log-Only Error", "Non-Critical Error", "RT Error" {
        # "Error - Display message in status indicator on panel.  If it's a critical error, shut down this VI with an 'Exit' message."
        n102 = case shown="Default" w274 {
          selector: w274 -> [_ w292]
          tunnel: ["UI Error" w292] -> w273
          frame Default {
          }
          frame "RT Error" {
          }
        }
        n103 = Variant To Data(error in=w288, type=errorcluster {"status"=FALSE, "code"=0, "source"=""} ("error constant"), Variant=w286) -> (data=w281:errorcluster, error out=w287:errorcluster)
        n104 = Unbundle By Name(w281) -> ("code"=w280:i32, "source"=w284:string)
        n105 = Format Date/Time String() -> (date/time string=w283:string)  [unwired: 3 in]
        n106 = Format Into String(format string="\n%s: %s %d - %s", w283, w273, w280, w284) -> (resulting string=w275:string)  [unwired: 2 in, 1 out]
        n107 = call "Enqueue Message.vi"("error in (no error)"=w287, "Message Data"=w275, "Message"="Update System Status", "Message Queue"=w278) -> ("error out"=w279:errorcluster, "dup Message Queue"=w277:refnum<queue>)  [unwired: 6 in]
        n108 = case shown="Default" w274 {
          tunnel: w279 -> [w293 w297]
          tunnel: w277 -> [_ w295]
          tunnel: [w293 w296] -> w289
          frame Default {
          }
          frame "Critical Error" {
            n109 = call "Enqueue Message.vi"("error in (no error)"=w297, "Message"="Exit", "Message Queue"=w295) -> ("error out"=w296:errorcluster)  [unwired: 7 in, 1 out]
          }
        }
      }
      frame "Update System Status" {
        # "#CodeRecommended - The code below ensures that the System Status string value does not become too large.  It uses the same maximum size as the RT error log to determine whether or not to remove the last half of the log string. Change this logic if you wish to maintain more/less of the information in the System Status string."
        # "Update System Status - Add a new string to the beginning of the System Status string on the UI."
        n110 = Variant To Data(error in=w309, type="", Variant=w306) -> (data=w303:string, error out=w307:errorcluster)
        n111 = local read "System Status"() -> (w301:string)
        n112 = global read "Global - Configuration Options.vi" "Error Log Max Size (bytes)"() -> (w299:i64)
        n113 = String Length(string=w301) -> (length=w302:i32)
        n114 = Greater?(x=w302, y=w299) -> (0:w300:bool)
        n115 = case shown="False" w300 {
          tunnel: w301 -> [w310 w314]
          tunnel: w299 -> [_ w313]
          tunnel: [w310 w315] -> w298
          frame False {
          }
          frame True {
            n116 = Divide(x=w313, y=i64 2) -> (x/y=w312:dbl)
            n117 = String Subset(string=w314, length (rest)=w312) -> (substring=w315:string)  [unwired: 1 in]
          }
        }
        n118 = Concatenate Strings(w303, w298) -> (→"System Status":string)
      }
      frame "Exit" {
        # "Close all connections"
        # "Stop Monitoring Loop"
        # "Stop Event Handling Loop"
        # "Release the UI Message queue reference"
        # "Stop UI Message Loop"
        # "Exit - Fire the User Event to stop the Event Handling Loop, and toggle the local variable to stop the Monitoring Loop.  This message alone causes all three loops to stop."
        n119 = local write "Connected?"(FALSE ("Connected?")) -> ()
        n120 = global write "Global - All UI Loop Stop.vi" "All UI Loop Stop"(TRUE ("Stop Monitoring Loop")) -> ()
        n121 = call "Fire User Event - Stop.vi"("User Event - Stop"=w325) -> ("error out"=w324:errorcluster)  [unwired: 10 in]
        n122 = Release Queue(queue=w321, error in (no error)=w326) -> (error out=w322:errorcluster)  [unwired: 1 in, 2 out]
        n123 = global read "Global - UI Stream and Variable Connections.vi" "UI Command Stream"() -> (w320:refnum<k21>)
        n124 = global read "Global - UI Stream and Variable Connections.vi" "RT Message Stream"() -> (w319:refnum<k21>)
        n125 = global read "Global - UI Stream and Variable Connections.vi" "Variable References"() -> (w316:T21)
        n126 = Destroy Stream Endpoint(11:w320) -> ()  [unwired: 1 in, 1 out]
        n127 = Destroy Stream Endpoint(11:w319) -> ()  [unwired: 1 in, 1 out]
        n128 = Merge Errors(w324, w322) -> (w327:errorcluster)
        n129 = call "Close Variable Connections.vi"("Variable References 2"=w316) -> ()  [unwired: 11 in]
      }
      frame "---Copy This Frame---" {
        # "Duplicate this frame when creating new messages.  Change this comment in the duplicated frame to describe this message."
        n130 = Merge Errors(w331) -> (w330:errorcluster)
      }
      frame "Update Tool Data" {
        # "Duplicate this frame when creating new messages.  Change this comment in the duplicated frame to describe this message."
        n131 = Variant To Data(type=path "" ("Tool Data File"), Variant=w340) -> (data=w332:path, error out=w334:errorcluster)  [unwired: 1 in]
        n132 = Build Path(name or relative path=w332) -> (appended path=w338:path)  [unwired: 1 in]
        n133 = Read from Text File(file (use dialog)=w338, error in=w334) -> (text=w335:string, error out=w337:errorcluster)  [unwired: 2 in, 2 out]
        n134 = Unbundle By Name(w337) -> ("status"=w336:bool)  [unwired: 1 out]
        n135 = case shown="False" w336 {
          tunnel: w335 -> [w344 _]
          tunnel: [w344 "Error"] -> w333
          frame False {
          }
          frame True {
          }
        }
        "Tool Data" <- w333
        n136 = Merge Errors(w343) -> (w342:errorcluster)
      }
      frame "Unsuccessful Connection" {
        # "Duplicate this frame when creating new messages.  Change this comment in the duplicated frame to describe this message."
        n137 = flat-sequence {
          tunnel: w350 -> [w353]
          tunnel: [w353] -> w349
          tunnel: w349 -> [w354]
          tunnel: w348 -> [w367]
          tunnel: [w366] -> w346
          tunnel: w347 -> [w365]
          frame #0 {
            n138 = local write "Connected?"(FALSE ("Connected?")) -> ()
          }
          frame #1 {
            w355 = 0
            n139 = Unbundle(w354) -> ("Switch to Safe State Ref"=w363:refnum<vi>, "Run Control Ref"=w362:refnum<vi>, "Stop Control Ref"=w361:refnum<vi>, "Update Control Configurations Ref"=w360:refnum<vi>, "Chatter Data Ref"=w359:refnum<vi>, "Max Acceleration Threshold Ref"=w358:refnum<vi>)
            n140 = property on="Controller Address" class="Str"("DisabledEnum"=w355) -> ()  [unwired: 2 in, 2 out]
            n141 = property on="Connect to Controller" class="Bool"("DisabledEnum"=w355) -> ()  [unwired: 2 in, 2 out]
            n142 = Build Array(w363, w362, w361, w360, w359, w358) -> (w357:refnum<vi>[])
            n143 = call "Set Enable State on Multiple Controls.vi"("Enable?"=FALSE, "Controls"=w357) -> ()  [unwired: 10 in]
          }
          frame #2 {
            n144 = Wait (ms)(milliseconds to wait=u32 1000) -> ()  [unwired: 1 out]
          }
          frame #3 {
            n145 = call "Enqueue Message.vi"("error in (no error)"=w367, "Message"="Connect", "Message Queue"=w365) -> ("error out"=w366:errorcluster)  [unwired: 7 in, 1 out]
          }
        }
        n146 = Merge Errors(w346) -> (w351:errorcluster)
      }
      frame Default {
        # "'Default' case only runs if there is a message that isn't defined in any of the other cases.  Output a programming error."
        n147 = Format Into String(format string="The invalid message string \"%s\" was received in the Message Handling Loop." ("Invalid Message Loop Message"), w373) -> (resulting string=w370:string)  [unwired: 2 in, 1 out]
        n148 = call <vilib>:"Error Cluster From Error Code.vi"("error message (\"\")"=w370, "error code (0)"=1) -> ("error out"=w371:errorcluster)  [unwired: 7 in]
      }
    }
    n149 = call "UI Error Handler - Message Handler.vi"("error in (no error)"=w64, "Message Queue"=w65) -> ()  [unwired: 9 in, 1 out]
    n150 = call <vilib>:"Clear Errors.vi"("error in (no error)"=w64) -> ("error out"=w63:errorcluster)  [unwired: 5 in, 1 out]
  }
  n151 = Tick Count (ms)() -> (millisecond timer value=w33:u32)
  n152 = while {
    tunnel: w45 -> [w375]
    tunnel: [w378] -> w55
    shift-right: [w376] -> w47
    shift-left: w53 -> [w377]
    stop <- w379 stop-if-true
    # "Event Handling Loop"
    n153 = event shown="[0] \"Connect to Controller\": Value Change" {
      selector: w377 -> [_ _ _ _ _ _ _ _]
      dyn-events: [_ _ _ _ _ _ _ _] -> w376
      timeout: _ -> [_ _ _ _ _ _ _ _]
      tunnel: [_ _ _ _ _ _ _ TRUE ("Discard?")] -> w380
      tunnel: w375 -> [w386 w389 w392 w395 w400 _ w405 _]
      tunnel: [w388 w391 w394 w397 w399 _ w408 _] -> w378
      tunnel: w375 -> [_ _ _ _ _ w404 _ _]
      event "Connect to Controller": Value Change {
        n154 = event-data() -> ()  [unwired: 1 in, 1 out]
        n155 = call "Enqueue Message.vi"("Message"="Connect", "Message Queue"=w386) -> ("error out"=w388:errorcluster)  [unwired: 8 in, 1 out]
      }
      event "Run Control": Value Change {
        n156 = event-data() -> ()  [unwired: 1 in, 1 out]
        n157 = call "Enqueue Message.vi"("Message"="Run Control", "Message Queue"=w389) -> ("error out"=w391:errorcluster)  [unwired: 8 in, 1 out]
      }
      event "Stop Control": Value Change {
        n158 = event-data() -> ()  [unwired: 1 in, 1 out]
        n159 = call "Enqueue Message.vi"("Message"="Stop Control", "Message Queue"=w392) -> ("error out"=w394:errorcluster)  [unwired: 8 in, 1 out]
      }
      event "Switch to Safe State": Value Change {
        n160 = event-data() -> ()  [unwired: 1 in, 1 out]
        n161 = call "Enqueue Message.vi"("Message"="Run Safe State", "Message Queue"=w395) -> ("error out"=w397:errorcluster)  [unwired: 8 in, 1 out]
      }
      event "Max Acceleration Threshold (g)": Value Change {
        n162 = event-data() -> ()  [unwired: 1 in, 1 out]
        n163 = call "Enqueue Message.vi"("Message Data"="Max Acceleration Threshold (g)", "Message"="Update Max Acceleration Threshold", "Message Queue"=w400) -> ("error out"=w399:errorcluster)  [unwired: 7 in, 1 out]
      }
      event "Tool Data File", "OK Button": Value Change {
        n164 = event-data() -> ()  [unwired: 1 in, 3 out]
        n165 = call "Enqueue Message.vi"("Message Data"="Tool Data File", "Message"="Update Tool Data", "Message Queue"=w404) -> ()  [unwired: 7 in, 2 out]
      }
      event "Exit": Value Change {
        w406 = TRUE  # Priority Message
        # "The UI Message Loop handles sending the Exit message to other loops."
        n166 = event-data() -> ()  [unwired: 1 in, 1 out]
        n167 = call "Enqueue Message.vi"("Priority Message? (F)"=w406, "Message"="Exit", "Message Queue"=w405) -> ("error out"=w408:errorcluster)  [unwired: 7 in, 1 out]
      }
      event User Event {
        # "The Message Handling Loop processed an \"Exit\" message, which fired this event to stop the Event Handling Loop."
        n168 = event-data() -> ()  [unwired: 1 in, 1 out]
      }
    }
    n169 = case shown="Error" w378 {
      tunnel: [w381 TRUE ("Discard?")] -> w379
      tunnel: w380 -> [w381 _]
      tunnel: w375 -> [_ w382]
      frame No Error {
      }
      frame Error {
        # "On error, send Exit message, and stop loop."
        n170 = call "Enqueue Message.vi"("Priority Message? (F)"=TRUE ("Discard?"), "Message"="Exit", "Message Queue"=w382) -> ()  [unwired: 7 in, 2 out]
      }
    }
  }
  n171 = call "mqttTXdataQueue.vi"("function"=mqttTXdataQueueFunction."init", "error in (no error)"="error in (no error)") -> ("error out"=w3:errorcluster)  [unwired: 12 in, 1 out]
  n172 = call "api_mqttInit.vi"("client"=w6, "broker"=T8 {"address"="amrcmtconnect.shef.ac.uk", "port"=1883, "connTimeout"=2000, "writeTimeout"=2000, "readTimeout"=2000, "subTimeout"=30000}, "connFlags"=T10 {"reserved"=FALSE, "clean session"=TRUE, "will flag"=TRUE, "willQOS"=enum."At most once", "will retain"=FALSE, "password"=FALSE, "user name"=FALSE}, "User Info"=T9 {"User Name"="User", "Password"="password"}, "error in (no error)"=w3) -> ("error out"=w4:errorcluster)  [unwired: 10 in]
  n173 = call "mqttConfigStore.vi"("function"=mqttConfigFunction."get", "error in (no error)"=w4) -> ("mqtt.lvclass out"=w11:refnum<class "mqtt.lvclass">, "error out"=w10:errorcluster)  [unwired: 12 in]
  n174 = call "mqttTCPIPserver.vi"("mqtt.lvclass"=w11, "error in (no error)"=w10) -> ()  [unwired: 12 in, 2 out]
  n175 = call "api_mqttConnect.vi"("error in (no error)"=w10) -> ("success"=→"success":bool, "connStatus"=→"connStatus 2":T3, "sessionPresent"=→"sessionPresent 2":bool, "error out"=w2:errorcluster)  [unwired: 11 in]
  n176 = while {
    tunnel: w45 -> [w415]
    tunnel: "milliseconds to wait" -> [w420]
    shift-right: [w416] -> _
    shift-left: w37 -> [w417]
    tunnel: w34 -> [w419]
    tunnel: w38 -> [w418]
    shift-right: [w412] -> _
    shift-left: w33 -> [w414]
    shift-right: [w410] -> _
    shift-left: w2 -> [w411]
    stop <- w422 stop-if-true
    # "Only read monitoring variables if the UI Main VI is connected to the RT target"
    # "Only the 'Exit' message in the UI Message Loop can stop the Monitoring Loop."
    # "Monitoring Loop"
    n177 = Tick Count (ms)() -> (millisecond timer value=w412:u32)
    n178 = Subtract(x=w412, y=w414) -> (x-y=→"Loop execution":u32)
    n179 = local read "Connected?"() -> (w421:bool)
    n180 = case shown="True" w421 {
      tunnel: w415 -> [_ w556]
      tunnel: w420 -> [w425 w552]
      tunnel: w417 -> [_ w540]
      tunnel: w419 -> [_ w539]
      tunnel: w418 -> [_ w538]
      tunnel: [w424 w537] -> w416
      tunnel: w417 -> [w424 w537]
      tunnel: w415 -> [_ w536]
      tunnel: w411 -> [w423 _]
      tunnel: w411 -> [_ w427]
      tunnel: [w423 w426] -> w410
      frame False {
        n181 = Wait (ms)(milliseconds to wait=w425) -> ()  [unwired: 1 out]
      }
      frame True {
        (unwired) 1 ("length")
        (unwired) sgl 0.0 ("Tolerance")
        # "Serialize the shared variable calls to simplify the scheduling performed by LabVIEW at runtime"
        n182 = Unbundle By Name("connMeta") -> ("qos"=w437:T2, "retain"=w436:bool, "duplicate"=w435:bool)
        n183 = feedback #1(u16 0) -> (w442:u16)
        n184 = Increment(x=w442) -> (x+1=w441:u16)
        "publishMessageID" <- w441
        n185 = feedback-in #1(w441) -> ()
        n186 = global read "Global - UI Stream and Variable Connections.vi" "Variable References"() -> (w554:T21)
        n187 = Unbundle By Name(w554) -> ("Current FPGA State"=w551:refnum<k21>, "Acceleration (grms)"=w548:refnum<k21>, "Acceleration Waveform"=w547:refnum<k21>, "Chatter"=w479:refnum<k21>, "tag acc"=w486:refnum<k21>, "tag video"=w485:refnum<k21>, "Free or Contiguous Memory"=w451:refnum<k21>, "DMA FIFO Overflow?"=w465:refnum<k21>, "CPU Usage"=w464:refnum<k21>, "Image Waveform"=w448:refnum<k21>)
        n188 = call "UI - Read Stream from RT.vi"("Message Queue"=w556) -> ("Message Received?"=w553:bool, "dup Message Queue"=w555:refnum<queue>)  [unwired: 8 in, 1 out]
        n189 = case shown="False" w553 {
          tunnel: w552 -> [w717 _]
          frame False {
            n190 = Wait Until Next ms Multiple(millisecond multiple=w717) -> ()  [unwired: 1 out]
          }
          frame True {
            # "If a message was received, immediately read again"
          }
        }
        n191 = shared-variable-read(w448) -> (w447:T26[])  [unwired: 1 in, 3 out]
        n192 = shared-variable-read(w551) -> (w550:errorcluster, w542:T25)  [unwired: 1 in, 2 out]
        "Current FPGA State" <- w542
        n193 = shared-variable-read(w548, w550) -> (w549:errorcluster, w480:dbl[])  [unwired: 2 out]
        n194 = shared-variable-read(w547, w549) -> (w530:errorcluster, w455:waveform(dbl)[], w453:timestamp)  [unwired: 1 out]
        n195 = shared-variable-read(w479, w530) -> (w487:errorcluster, w529:bool[])  [unwired: 2 out]
        n196 = shared-variable-read(w486, w487) -> (w484:errorcluster, w446:string)  [unwired: 2 out]
        "tag acc" <- w446
        "string" <- w446
        n197 = shared-variable-read(w485, w484) -> (w483:errorcluster, w450:string)  [unwired: 2 out]
        "tag spike" <- w450
        n198 = Boolean To (0,1)(Boolean=w529) -> (0, 1=w473:i16[])
        n199 = for {
          tunnel: w540 -> [w585] mode=indexing
          shift-right: [w587] -> w535
          shift-left: w483 -> [w586]
          tunnel: [w579] -> w513 mode=indexing
          tunnel: [w584] -> w527
          tunnel: w536 -> [w584]
          tunnel: w538 -> [w583]
          tunnel: w539 -> [w582]
          tunnel: [w580] -> w482
          tunnel: [w581] -> w476
          n200 = case "Message Cases" shown="\"Machine Data\"" w585 {
            tunnel: w586 -> [w594 w599 w606 w613 w621 w628 w635 w642 w649 w656 w663 w670 w677 w684 w691 w698 w703]
            tunnel: [w593 w598 w605 w611 w621 w628 w635 w642 w649 w656 w663 w670 w677 w684 w691 w698 w709] -> w587
            tunnel: [w588 w597 w602 w607 w616 w623 w630 w637 w644 w651 w659 w665 w673 w679 w686 w695 w699] -> w579
            tunnel: w583 -> [w590 w596 w604 w612 w617 w624 w631 w638 w645 w652 w657 w669 w671 w683 w687 w693 _]
            tunnel: w582 -> [_ _ _ _ _ _ _ _ _ _ _ _ _ _ _ _ w702]
            tunnel: [FALSE ("Triggger G1,G2, or G3") FALSE ("Triggger G1,G2, or G3") FALSE ("Triggger G1,G2, or G3") FALSE ("Triggger G1,G2, or G3") FALSE ("Triggger G1,G2, or G3") FALSE ("Triggger G1,G2, or G3") FALSE ("Triggger G1,G2, or G3") FALSE ("Triggger G1,G2, or G3") FALSE ("Triggger G1,G2, or G3") FALSE ("Triggger G1,G2, or G3") FALSE ("Triggger G1,G2, or G3") FALSE ("Triggger G1,G2, or G3") FALSE ("Triggger G1,G2, or G3") FALSE ("Triggger G1,G2, or G3") FALSE ("Triggger G1,G2, or G3") FALSE ("Triggger G1,G2, or G3") w708] -> w580
            tunnel: [_ _ _ _ _ _ _ _ _ _ _ _ _ _ _ _ w700] -> w581
            frame "Spindle Load" {
              # "maximum spindle power"
              # "Action 1 - Send an \"Update Display\" message indicating which button was pressed. Note that a string is sent as the Message Data along with the \"Update Display\" message."
              n201 = call "read_data_spindle_load_mt_connect (SubVI).vi"("error in (no error)"=w594, "URL"=w590) -> ("error out"=w593:errorcluster, "number"=w591:dbl[])  [unwired: 8 in]
              n202 = Multiply(x=1, y=w591) -> (x*y=w588:dbl[])
              "Spindle Load" <- w588
            }
            frame "Spindle Speed" {
              # "Action 2 - Send an \"Update Display\" message indicating which button was pressed. Note that a string is sent as the Message Data along with the \"Update Display\" message."
              n203 = call "read_data_speed_mt_connect (SubVI).vi"("error in (no error)"=w599, "URL"=w596) -> ("error out"=w598:errorcluster, "number"=w597:dbl[])  [unwired: 8 in]
            }
            frame "Feed Rate", Default {
              n204 = call "read_data_feed_mt_connect (SubVI).vi"("error in (no error)"=w606, "URL"=w604) -> ("error out"=w605:errorcluster, "appended array"=w602:dbl[])  [unwired: 8 in]
              n205 = Index Array(array=w602, index=0) -> (element=→"Feed":dbl)
            }
            frame "Position I" {
              n206 = call "read_data_linear_position_mt_connect (SubVI).vi"("error in (no error)"=w613, "URL"=w612) -> ("error out"=w611:errorcluster, "I, J,K,X, Y,Z"=w609:dbl[])  [unwired: 8 in]
              n207 = Index Array(array=w609, index=0) -> (element=w608:dbl)
              n208 = Build Array(w608) -> (w607:dbl[])
            }
            frame "Position J" {
              n209 = call "read_data_linear_position_mt_connect (SubVI).vi"("URL"=w617) -> ("I, J,K,X, Y,Z"=w619:dbl[])  [unwired: 9 in, 1 out]
              n210 = Index Array(array=w619, index=1) -> (element=w618:dbl)
              n211 = Build Array(w618) -> (w616:dbl[])
            }
            frame "Position K" {
              n212 = call "read_data_linear_position_mt_connect (SubVI).vi"("URL"=w624) -> ("I, J,K,X, Y,Z"=w626:dbl[])  [unwired: 9 in, 1 out]
              n213 = Index Array(array=w626, index=2) -> (element=w625:dbl)
              n214 = Build Array(w625) -> (w623:dbl[])
            }
            frame "Position X" {
              n215 = call "read_data_linear_position_mt_connect (SubVI).vi"("URL"=w631) -> ("I, J,K,X, Y,Z"=w633:dbl[])  [unwired: 9 in, 1 out]
              n216 = Index Array(array=w633, index=3) -> (element=w632:dbl)
              n217 = Build Array(w632) -> (w630:dbl[])
            }
            frame "Position Y" {
              n218 = call "read_data_linear_position_mt_connect (SubVI).vi"("URL"=w638) -> ("I, J,K,X, Y,Z"=w640:dbl[])  [unwired: 9 in, 1 out]
              n219 = Index Array(array=w640, index=4) -> (element=w639:dbl)
              n220 = Build Array(w639) -> (w637:dbl[])
            }
            frame "Position Z" {
              n221 = call "read_data_linear_position_mt_connect (SubVI).vi"("URL"=w645) -> ("I, J,K,X, Y,Z"=w647:dbl[])  [unwired: 9 in, 1 out]
              n222 = Index Array(array=w647, index=5) -> (element=w646:dbl)
              n223 = Build Array(w646) -> (w644:dbl[])
            }
            frame "Position A" {
              n224 = call "read_data_linear_angle_mt_connect (SubVI).vi"("URL"=w652) -> ("I, J,K,X, Y,Z"=w654:dbl[])  [unwired: 9 in, 1 out]
              n225 = Index Array(array=w654, index=0) -> (element=w653:dbl)
              n226 = Build Array(w653) -> (w651:dbl[])
            }
            frame "Position B" {
              n227 = call "read_data_linear_angle_mt_connect (SubVI).vi"("URL"=w657) -> ("I, J,K,X, Y,Z"=w661:dbl[])  [unwired: 9 in, 1 out]
              n228 = Index Array(array=w661, index=1) -> (element=w660:dbl)
              n229 = Build Array(w660) -> (w659:dbl[])
            }
            frame "Xload" {
              n230 = call "read_data_linear_loadX_mt_connect (SubVI).vi"("URL"=w669) -> ("I, J,K,X, Y,Z"=w667:dbl[])  [unwired: 9 in, 1 out]
              n231 = Index Array(array=w667, index=0) -> (element=w666:dbl)
              n232 = Build Array(w666) -> (w665:dbl[])
            }
            frame "Yload" {
              n233 = call "read_data_linear_loadX_mt_connect (SubVI).vi"("URL"=w671) -> ("I, J,K,X, Y,Z"=w675:dbl[])  [unwired: 9 in, 1 out]
              n234 = Index Array(array=w675, index=1) -> (element=w674:dbl)
              n235 = Build Array(w674) -> (w673:dbl[])
            }
            frame "Zload" {
              n236 = call "read_data_linear_loadX_mt_connect (SubVI).vi"("URL"=w683) -> ("I, J,K,X, Y,Z"=w680:dbl[])  [unwired: 9 in, 1 out]
              n237 = Index Array(array=w680, index=2) -> (element=w681:dbl)
              n238 = Build Array(w681) -> (w679:dbl[])
            }
            frame "Aload" {
              n239 = call "read_data_angle_loadmt_connect (SubVI).vi"("URL"=w687) -> ("I, J,K,X, Y,Z"=w689:dbl[])  [unwired: 9 in, 1 out]
              n240 = Index Array(array=w689, index=0) -> (element=w688:dbl)
              n241 = Build Array(w688) -> (w686:dbl[])
            }
            frame "Bload" {
              n242 = call "read_data_angle_loadmt_connect (SubVI).vi"("URL"=w693) -> ("I, J,K,X, Y,Z"=w692:dbl[])  [unwired: 9 in, 1 out]
              n243 = Index Array(array=w692, index=1) -> (element=w697:dbl)
              n244 = Build Array(w697) -> (w695:dbl[])
            }
            frame "Machine Data" {
              n245 = call "read_machine_parameters_mt_connect (SubVI).vi"("URL 2"=w702, "error in (no error) 3"=w703) -> ("error out 3"=w701:errorcluster, "Machine Data"=w700:T22)  [unwired: 7 in]
              n246 = Unbundle By Name(w700) -> ("Block of code being executed"=w710:string)
              "Block of code being executed" <- w710
              n247 = Unbundle By Name(w700) -> ("Tool_id"=→"Tool id":string, "Program Name"=w707:string)
              "Program Name" <- w707
              n248 = Decimal String To Number(string=w707) -> (number=w706:i32)  [unwired: 2 in, 1 out]
              n249 = call "check_G1_G2_G3.vi"("current line"=w710, "error in (no error)"=w701) -> ("Triggger G1,G2, or G3"=w708:bool, "error out (no error)"=w709:errorcluster)  [unwired: 7 in]
              n250 = To Double Precision Float(number=w706) -> (double precision float=w705:dbl)
              n251 = Build Array(w705) -> (w699:dbl[])
            }
          }
        }
        n252 = Or(x=w482, y="Save?") -> (x .or. y?=w458:bool)
        n253 = Equal?(x=w542, y=FPGA_state."Safe State") -> (x = y?=w544:bool)
        n254 = feedback #2(timestamp(0 s since 1904-01-01)) -> (w546:timestamp)
        n255 = feedback-in #2(w453) -> ()
        n256 = case shown="True" w544 {
          frame False {
            n257 = property on="Run Control" class="Bool"("DisabledEnum"=T12."Disabled and Grayed Out" ("Disabled")) -> ()  [unwired: 2 in, 2 out]
            n258 = property on="Stop Control" class="Bool"("DisabledEnum"=T12."Enabled" ("Disabled")) -> ()  [unwired: 2 in, 2 out]
          }
          frame True {
            n259 = property on="Run Control" class="Bool"("DisabledEnum"=T12."Enabled" ("Disabled")) -> ()  [unwired: 2 in, 2 out]
            n260 = property on="Stop Control" class="Bool"("DisabledEnum"=T12."Disabled and Grayed Out" ("Disabled")) -> ()  [unwired: 2 in, 2 out]
          }
        }
        n261 = Array Subset(array=w480, index=0, length=3) -> (w444:dbl[])
        n262 = Equal?(x=w453, y=w546) -> (x = y?=w481:bool)
        n263 = Array To Cluster(array=w444) -> (cluster=→"ACC  (grms)":cluster{"[0]":dbl, "[1]":dbl, "[2]":dbl})
        n264 = control-ref of="STC Starrag"() -> (w506:refnum<vi>)
        n265 = shared-variable-read(w451) -> (→"Free Physical Memory or Largest Contiguous Memory (bytes)":dbl)  [unwired: 1 in, 3 out]
        n266 = case shown="True" w481 {
          tunnel: w455 -> [_ w716]
          tunnel: w455 -> [w715 _]
          tunnel: [w715 w716] -> w452
          frame False {
            "Raw Waveform" <- w715
          }
          frame True {
          }
        }
        n267 = property on="Property Node" class="Bool (strict)"(reference=w506) -> ("Colors [4]"=w500:cluster{u32, u32}[])  [unwired: 1 in, 2 out]
        n268 = shared-variable-read(w465) -> (w471:errorcluster, →"DMA FIFO Overflow?":bool)  [unwired: 1 in, 2 out]
        n269 = shared-variable-read(w464, w471) -> (w470:T27)  [unwired: 3 out]
        n270 = for {
          tunnel: w470 -> [w562] mode=indexing
          tunnel: [w561] -> w469 mode=indexing
          n271 = Unbundle By Name(w562) -> ("Total (%)"=w561:dbl)
        }
        n272 = Bundle By Name(cluster=T24 {"Magnitude threshold"=0.0, "Tolerance"=0.0} ("Limits"), "Magnitude threshold"=sgl 0.00015, "Tolerance"=sgl 2.0) -> (w519:T24)
        n273 = Array Size(array=w469) -> (size(s)=w468:i32)
        n274 = Reshape Array(w469, 1 ("dimension size"), w468) -> (→"CPU Usage (%)":dbl[][])
        n275 = Index Array(array=w500, index=2) -> (element=w502:cluster{u32, u32})
        n276 = Array Subset(array=w444, index=3, length=3) -> (w489:dbl[])
        n277 = Get Date/Time In Seconds() -> (seconds since 1Jan1904=w541:timestamp)
        n278 = Index Array(array=w513, index (row)=1, index (col)=0 ("disabled index (col)")) -> (element=w514:dbl)
        "RPM" <- w514
        n279 = Bundle By Name(cluster=cluster{"rpm":sgl} {"rpm"=0.0} ("Cutting data"), "rpm"=w514) -> (w521:cluster{"rpm":sgl})
        n280 = Build Array(w444) -> (w532:dbl[][])
        n281 = Array To Cluster(array=w489) -> (cluster=→"Force (grms)":T7)
        n282 = Transpose 2D Array(2D array=w532) -> (transposed array=w531:dbl[][])
        n283 = Or(x="Save?", y=w482) -> (x .or. y?=w478:bool)
        n284 = Insert Into Array(array=w513, new element=w531) -> (w445:dbl[][])  [unwired: 2 in]
        n285 = case shown="False" w478 {
          tunnel: w446 -> [_ w567]
          tunnel: [w565 w569] -> w477
          tunnel: w476 -> [w566 w568]
          tunnel: w450 -> [_ _]
          frame False {
            n286 = Bundle By Name(cluster=w566, "path_position"="Unavailable" ("Tool_id"), "Xload"="Unavailable" ("Tool_id")) -> (w565:T22)
          }
          frame True {
            n287 = Bundle By Name(cluster=w568, "path_position"=w567, "Xload"=w567) -> (w569:T22)
          }
        }
        n288 = Bundle("seconds since 1Jan1904"=w541, "appended array"=w445, "Machine Data"=w477) -> (w428:T28)  [unwired: 1 in]
        n289 = Unbundle(w428) -> ("seconds since 1Jan1904"=w434:timestamp, "appended array"=w432:dbl[][], "Machine Data"=w433:T22)
        n290 = Index Array(array=w432, index (col)=0 ("disabled index (col)")) -> (element=w430:dbl[])  [unwired: 1 in]
        n291 = call "MQTT_10Hz.vi"("data 2"=w430, "Machine Data"=w433, "current time 2"=w434) -> ("JSON string"=w429:string)  [unwired: 8 in]
        n292 = call "api_mqttPublish.vi"("topic"="topic", "value"=w429, "QoS (At most once)"=w437, "messageID"=w441, "error in (no error)"=w427, "retain(F)"=w436, "duplicate(F)"=w435) -> ("success"=→"publishSuccess":bool, "error out"=w426:errorcluster)  [unwired: 7 in]
        n293 = To Variant(anything=w428) -> (Variant=w533:variant)
        n294 = Unbundle By Name(w476) -> ("Program status"=w461:string)
        n295 = case shown="\"INTERRUPTED\"" w461 {
          tunnel: [u32 16723242 u32 6618880 u32 16449369 u32 16449369 u32 16449369] -> w499
          frame "Stopped", Default {
          }
          frame "ACTIVE" {
          }
          frame "INTERRUPTED" {
          }
          frame "FEED_HOLD" {
          }
          frame "READY" {
          }
        }
        n296 = Bundle(cluster=w502, w499) -> (w503:cluster{u32, u32})  [unwired: 1 in]
        n297 = Insert Into Array(array=w500, index=0, new element #1=w503, new element #2=w503, new element #3=w503, new element #4=w503) -> (w501:cluster{u32, u32}[])
        n298 = property on="Property Node" class="Bool (strict)"(reference=w506, "Colors [4]"=w501) -> ()  [unwired: 1 in, 2 out]
        n299 = Equal?(x=w461, y="ACTIVE") -> (x = y?=w460:bool)
        n300 = Index Array(array=w513, index (row)=0, index (col)=0 ("disabled index (col)")) -> (element=w510:dbl)
        n301 = Greater?(x=w510, y="In-cut Power Threshold") -> (0:w495:bool)
        n302 = And(x=w495, y=w478) -> (x .and. y?=w494:bool)
        n303 = case shown="False" w494 {
          tunnel: w473 -> [_ w576]
          tunnel: [w575 w576] -> w498
          tunnel: i16[] [0, 0, 0] ("0, 1") -> [w575 _]
          frame False {
          }
          frame True {
          }
        }
        n304 = Not Equal To 0?(x=w498) -> (x != 0?=w497:bool[])
        n305 = Or Array Elements(Boolean array=w497) -> (logical OR=→"Chatter?":bool)
        n306 = case shown="True" w460 {
          tunnel: [sgl 0.0 ("Tolerance") sgl 1.0 ("Tolerance")] -> w459
          tunnel: [FALSE TRUE] -> w457
          frame False {
          }
          frame True {
          }
        }
        n307 = Or(x=w458, y=w457) -> (x .or. y?=w456:bool)
        "x .or. y?" <- w456
        n308 = Bundle By Name(cluster=cluster{"Number of teeth":sgl} {"Number of teeth"=0.0} ("Tool data"), "Number of teeth"=w459) -> (w523:cluster{"Number of teeth":sgl})
        n309 = Bundle By Name(cluster=cluster{"G1 ":bool} {"G1 "=FALSE} ("G1 status"), "G1"=w456) -> (w449:cluster{"G1 ":bool})
        "output cluster" <- w449
        n310 = Bundle By Name(cluster=T17 {"Tool data"={"Number of teeth"=2.0}, "Cutting data"={"rpm"=9898.0}, "Limits"={"Magnitude threshold"=0.0, "Tolerance"=1.0}, "G1 status"={"G1 "=FALSE}} ("Chatter Data"), "Tool data"=w523, "Cutting data"=w521, "Limits"=w519, "G1 status"=w449) -> (w515:T17)
        n311 = call "Enqueue Message.vi"("Message Data"=w515, "Message"="Update Control Configuration", "Message Queue"=w527) -> ()  [unwired: 7 in, 2 out]
        n312 = case shown="False" w478 {
          tunnel: ["Plot" ("Message") "Plot and Save" ("Message")] -> w534
          tunnel: w452 -> [_ _]
          tunnel: w447 -> [_ _]
          tunnel: w450 -> [_ _]
          frame False {
          }
          frame True {
            (unwired) errorcluster {"status"=FALSE, "code"=0, "source"=""} ("error out")
          }
        }
        n313 = call "Enqueue Message.vi"("error in (no error)"=w535, "Message Data"=w533, "Message"=w534, "Message Queue"=w527) -> ("error out"=w507:errorcluster)  [unwired: 6 in, 1 out]
        n314 = call "UI Error Handler - Monitoring.vi"("error in (no error)"=w507, "Message Queue"=w555) -> ()  [unwired: 9 in, 1 out]
      }
    }
    n315 = global read "Global - All UI Loop Stop.vi" "All UI Loop Stop"() -> (w422:bool)
  }
  n316 = Unregister For Events(event registration refnum=w47, error in=w55) -> (error out=w48:errorcluster)
  n317 = Merge Errors(w48, w56) -> (w54:errorcluster)
  n318 = call "Destroy User Event - Stop.vi"("error in (no error)"=w54, "User Event - Stop"=w52) -> ("error out"=w46:errorcluster)  [unwired: 9 in]
  n319 = call <vilib>:"Simple Error Handler.vi"("error in (no error)"=w46) -> ()  [unwired: 4 in, 5 out]
